vi "FrontPanel-20220513-backup.vi"() -> ()   [LabVIEW 2019]
doc: "This VI controls the blindpanel type GHS-2T-1T-700 for a CryoFree DR. Automatization control is embedded in the blindpanel. Keys can be manipulated from within this VI."
uses:
  1. Sources/Lib/Lib.llb/ErrCodeStatusLkup.vi
  1. Sources/Lib/Lib.llb/Pfeiffer Vacuum.lvlib
  1. Sources/Lib/Lib.llb/MView.lvlib
  1. Sources/Lib/Lib.llb/Busy PopUp.lvlib
  shared/FP-TC-Shared/FP-TC-Shared.lvclass
panel:
  out "VIRef":T1 {"Array DataType" format="%.0x"; "WaveForm Type" format="%.0x"; "RefNum Type" format="%.0x"; "DataType" format="%.0x"}
  out "ControlNames":string[](array[string])
  in  "Toolbar":enum32{"Page 1", "Page 2"}(tab)
  in  "Load config":bool
  in  "Save config":bool
  in  "Start":bool
  in  "Stop":bool
  out "V":string
  out "PT2 Data":dbl[](array[numeric])
  in  "Restart PT on Error?":bool
  in  "Attempts":u16=6
  in  "Time delay":u16=60 format="%.0f s"
  out "Error Log":string[][](table)
  in  "Error panel":enum32{"Page 1"}(tab)
  out "PT2 error":errorcluster
  out "MG error":errorcluster
  out "PT1 error":errorcluster
  out "FP error":errorcluster
  out "PT1 Data":dbl[](array[numeric])
  in  "Main Panel":enum32{"Page 1", "Page 2"}(tab)
  out "PC":sgl
  out "P1":sgl format="%.1f"
  out "P2":sgl format="%.1f"
  out "P3":sgl format="%.1f"
  out "P4":sgl format="%.1f"
  out "P5":sgl format="%.1f"
  out "P6":sgl format="%.1f"
  out "P7":sgl format="%.1f"
  out "Flow":sgl format="%#_4f"
  out "P5 alarm":bool
  out "Pstill (P8)":dbl format="%.1e"
  in  "Main Panel":T2(tab)
  out "String 2":string
  out "String 4":string
  out "String":string
  out "String 3":string
  out "Mode":u16(ring) items=["AUTO MODE OFF", "START", "CONDENSING 3He", "CONDENSING 4He", "NORMAL CIRCULATION", "RECOVERY OF THE MIXTURE", "RECOVERY: BLOCKAGE OR OVERPRESSURE"]
  out "FLOW":sgl format="%#_3f"
  out "P5":sgl
  out "P4":sgl
  out "P3":sgl
  out "P1":sgl
  out "P2":sgl
  out "3He":sgl(slide) min=0 max=2 scale=0.0..2000.0 scale format="%.2f"
  out "4He":sgl(slide) min=0 max=2 scale=0.0..2000.0 scale format="%.2f"
  out "Panel ID":string
  in  "FP type":enum32{"OLD", "NEW"}(tab)
  in  "Buttons":T3
  out "LEDs":T4
  in  "Buttons 2":T3
  out "LEDs 2":T5
  out "PC":sgl
  in  "PT Start 2":bool
  in  "PT_stop 2":bool
  in  "PT2 Plots Select":T6
  out "PT2 Status":cluster{"Time":dbl[], "Value":dbl[]}[](graph)
  in  "PT_ResetValues 2":bool
  out "PT Error Code 2":i32 caption="PT Error Code"
  out "PT Error 2":string="NO ERROR" caption="PT Error"
  out "P High":cluster{dbl, dbl, dbl, dbl}(slide) scale=150.0..450.0
  out "P Low":cluster{dbl, dbl, dbl, dbl}(slide) scale=0.0..300.0
  out "P_avg 2":cluster{"Low":dbl, "High":dbl} caption="Average pressure"
  out "Helium":cluster{dbl, dbl, dbl, dbl}(slide) scale=0.0..95.0
  out "Water In":cluster{dbl, dbl, dbl, dbl}(slide) scale=0.0..35.0
  out "Water Out":cluster{dbl, dbl, dbl, dbl}(slide) scale=0.0..60.0
  out "PT Status":u16(ring) items=["Compressor OFF", "Compressor ON", ""]
  out "Motor":cluster{dbl, dbl}(slide) scale=0.0..30.0
  out "Oil":cluster{dbl, dbl, dbl, dbl}(slide) scale=0.0..60.0
  in  "PT1 Plots Select":T6
  out "PT1 Status 2":cluster{"Time":dbl[], "Value":dbl[]}[](graph)
  out "P Low":cluster{dbl, dbl, dbl, dbl}(slide) scale=0.0..300.0
  out "P High":cluster{dbl, dbl, dbl, dbl}(slide) scale=150.0..450.0
  out "P_avg":cluster{"Low":dbl, "High":dbl} caption="Average pressure"
  out "Motor":cluster{dbl, dbl}(slide) scale=0.0..30.0
  out "Oil":cluster{dbl, dbl, dbl, dbl}(slide) scale=0.0..60.0
  out "Helium":cluster{dbl, dbl, dbl, dbl}(slide) scale=0.0..95.0
  out "Water Out":cluster{dbl, dbl, dbl, dbl}(slide) scale=0.0..60.0
  out "Water In":cluster{dbl, dbl, dbl, dbl}(slide) scale=0.0..35.0
  out "PT Error Code":i32
  out "PT Error":string="NO ERROR"
  in  "PT_ResetValues":bool
  in  "PT Start":bool
  in  "PT_stop":bool
  out "PT Status":u16(ring) items=["Compressor OFF", "Compressor ON", ""]
  in  "MG Plots Select":T6
  in  "FP Plots Select":T6
  out "MaxiGauge":cluster{"Time":dbl[], "Value":dbl[]}[](graph)
  out "Front Panel":cluster{"Time":dbl[], "Value":dbl[]}[](graph)
  in  "Boolean 2":bool
  out "PT2 port":u16
  out "PT1 port":u16
  out "MG port":refnum<visa-resource-name>="COM4" caption="Port number"
  out "FP port":refnum<visa-resource-name>="COM3" caption="Port number"
  out "ForceSave":bool
  in  "Button":u8
  out "SetControl":T7
  in  "S2":enum32{"Page 1"}(tab)
  in  "Reset Error 2":bool
  in  "S1":enum32{"Page 1"}(tab)
  in  "Reset Error":bool
  out "Cur Path":path
  in  "Side Panel":enum32{"Main", "Settings", "Advanced"}(tab)=enum."Settings"
  out "Maxigauge ID":string caption="ID"
  out "Panel response":string
  out "Sensors Status":T8={"String 8"="OK", "String 9"="OK", "String 10"="OK", "String 11"="OK", "String 12"="OK", "String 13"="OK"}
  in  "ADC scaling":T9={"P1"=2500.0, "P2"=2500.0, "P3"=2500.0, "P4"=2500.0, "P5"=2500.0, "P6"=2500.0, "P7"=2500.0, "Flow meter"=682.0, "PC"=10000.0} caption="Front panel ADC scaling factors" {"Flow meter" format="%#.4f"}
  in  "REC Settings":T10={"P6 low"=20, "P6 high"=1000, "P7 low"=20}
  in  "NCP5B Settings":cluster{"P6 low":u16}={"P6 low"=20}
  in  "NCP5 Settings":T10={"P6 low"=20, "P6 high"=1000, "P7 low"=20}
  in  "S1&2 Settings":cluster{"Enum":enum16{"OFF", "ON"}}
  in  "P5 Settings":cluster{"P6 low":u16, "P6 high":u16}={"P6 low"=20, "P6 high"=1000}
  out "REC limits":T11={"P5 warn"=20, "P5 rec"=20, "P5 res"=20}
  out "NCP5B limits":cluster{"P5 NC4":u16}={"P5 NC4"=20}
  out "NCP5 limits":T12={"P5 NC1"=20, "P5 NC2"=20, "P5 NC3"=20}
  out "S1&2 limits":cluster{"S1&S2":enum16{"OFF", "ON"}}
  out "P5 limits":cluster{"P5 C1":u16, "P5 C2":u16}={"P5 C1"=20, "P5 C2"=20}
  in  "P6&7 Settings":T13={"P6 low"=20, "P6 high"=1600, "P7 low"=20, "P7 high"=1610}
  out "P6&7 limits":T13={"P6 low"=20, "P6 high"=20, "P7 low"=20, "P7 high"=20}
  in  "SET VALUES":bool
  out "MG pressures":T14 {"Channel 1" format="%-7.2e mbar"; "Channel 1" format="%-7.2e mbar"; "Channel 1" format="%-7.2e mbar"; "Channel 1" format="%-7.2e mbar"; "Channel 1" format="%-7.2e mbar"; "Channel 1" format="%-7.2e mbar"}
  out "Cluster":T15={"String 2"="\"\"", "String 3"="", "String 4"="", "String 5"="", "String 6"="", "String 7"=""}
  in  "Log Options":T16={"Plot data "=TRUE, "Every1"=1.0, "Save to log"=TRUE, "Every  2"=1.0, "AVS_Path 2"=path "C:/LC Data/Data", "AVS_FName"="logFP", "Filename suffix"="_%Y-%m-%d-%H-%M-%S", "NewFevery"=7, "Time Units"=enum."Days", "Date Format"="%Y-%m-%d %H:%M:%S", "Averages"=4} caption="Data Logging \nOptions" {"Every  2" format="%#_g min"; "Every1" format="%#_g min"}
  in  "Configuration":T17={"FP port number"="COM3", "MG port number"="COM4", "PT1 Enabled?"=FALSE, "MG  channel P8"=65535, "Stop auto recovery if still is empty"=FALSE, "PT1 port number"="COM2", "MG Enabled?"=TRUE, "PT1 Address"=16, "S1 Enabled?"=FALSE, "S1 port"="COM2", "S2 Enabled?"=FALSE, "S2 port"="COM2", "Device address S1"=1, "Device address S2"=2, "PT1 Bauds"=115200, "PT2 Enabled?"=FALSE, "PT2 port number"="COM2", "PT2 Address"=16, "PT2 Bauds"=115200, "FP baud rate"=9600} {"PT2 Address" min=16 max=126 step=1; "MG  channel P8" items=["Channel 1", "Channel 2", "Channel 3", "Channel 4", "Channel 5", "Channel 6"]; "PT1 Address" min=16 max=126 step=1}
  in  "Type":enum32{"Wet", "CF"}(radio)=enum."CF"
  in  "Panel Layout":enum32{"OLD", "NEW"}(ring)=enum."NEW"
  out "RAW ADC Values 2":dbl[](array[numeric]) caption="Converted ADC Values"
  in  "SendCMD":bool caption="Send"
  out "Response":string
  in  "Command":string
  out "SP reached? 2":bool
  in  "Cond1":bool
  in  "Delay Time":u32=30 caption="For a time delay of" format="%.0f min"
  in  "MG  channel":u16(ring)=65535 caption="MaxiGauge" items=["Channel 1", "Channel 2", "Channel 3", "Channel 4", "Channel 5", "Channel 6"]
  out "SP reached? 3":bool
  in  "P threshold":dbl=0.0005 caption="<" format="%#_2g mbar"
  in  "Cond2":bool
  out "SP reached?":bool
  out "Delay Timer":u32=10 caption="Timer" format="%<%M:%S>t"
  in  "EnableAutoCond":bool caption="Start"
  out "VI path":string
  out "RAW ADC Values":i32[](array[numeric])
  in  "Autoconf":bool caption="Autoconfigure"
  out "MG Data":dbl[](array[numeric]) format="%.3e"
  out "FP Data":sgl[](array[numeric]) format="%.2f"
  out "FP Status bits":u32[](array[numeric])
  out "Attempts Counter":u16
  # "Error log"
  # "Front panel status"
  # "MaxiGauge status"
  # "Pulse Tube 1 status"
  # "Pulse Tube 2 status"
  # "Leiden Cryogenics"
  # "to \nair"
  # "N.C."
  # "from\novc"
  # "from\nivc"
  # "from still"
  # "to 3He\nin-1"
  # "to 3He\nin-2"
  # "P8"
  # "AUX 1"
  # "BYPASS"
  # "MIXTURE\nCOMPRESSOR"
  # "M2"
  # "P6"
  # "M3"
  # "M1"
  # "AUX PORT-1"
  # "P7"
  # "TRAP"
  # "AUX TRAP"
  # "To \nAir"
  # "From\nIVC"
  # "From Still"
  # "To 3He\nin-1"
  # "To 3He\nin-2"
  # "To \nAir"
  # "N.C."
  # "from\novc"
  # "from\nivc"
  # "from still"
  # "to 3He\nin-1"
  # "to 3He\nin-2"
  # "Leiden Cryogenics"
  # "to \nair"
  # "N.C."
  # "from\novc"
  # "from\nivc"
  # "from still"
  # "to 3He\nin-1"
  # "to 3He\nin-2"
  # "P8"
  # "M2"
  # "P6"
  # "M3"
  # "TRAP"
  # "AUX TRAP"
  # "M1"
  # "AUX PORT-1"
  # "P7"
  # "AUX 1"
  # "To \nAir"
  # "From\nIVC"
  # "From Still"
  # "To 3He\nin-1"
  # "to 3He\nin-1"
  # "To 3He\nin-2"
  # "to \nair"
  # "N.C."
  # "from\novc"
  # "from\nivc"
  # "from still"
  # "to 3He\nin-2"
  # "Pulse Tube 1"
  # "Pulse Tube 2"
  # "Front Panel"
  # "MaxiGauge"
  # "Turbo2 (S2)"
  # "Turbo1 (S1)"
  # "MaxiGauge"
  # "#"
  # "NAME"
  # "PRESSURE"
  # "STATUS"
  # "1"
  # "2"
  # "3"
  # "4"
  # "5"
  # "6"
  # "Automatic mode pressure limits"
  # "Warning: These values influence the operation of the GHS in automatic mode. Please refer to the operation manual and consult with Leiden Cryogenics before changing them."
  # "NAME"
  # "FW"
  # "NEW"
  # "DESCRIPTION"
  # "Stop condensing 4He"
  # "Stop recovering 4He"
  # "Stop condensing 3He"
  # "Stop recovering 3He"
  # "Condensing->open 12"
  # "Condensing->close 9/12"
  # "Condensing->run S1&S2"
  # "NC->open second line"
  # "NC->start MC"
  # "NC->open aux. trap"
  # "NC->stop MC, close 7"
  # "All->P5 alarm"
  # "All->switch to recovery"
  # "All->reset"
  # "Front panel ADC scaling factors"
  # "Data Logging and Plotting"
  # "Front Panel"
  # "MaxiGauge"
  # "Pulse Tube 1"
  # "Pulse Tube 2"
  # "Turbo 1 (S1) (Pfeiffer HiPACE only)"
  # "Turbo2 (S2) (Pfeiffer HiPACE only)"
  # "Automatic condensing"
  # "Start condensing when"
  # "and wait"
  # "Send command to Front Panel"
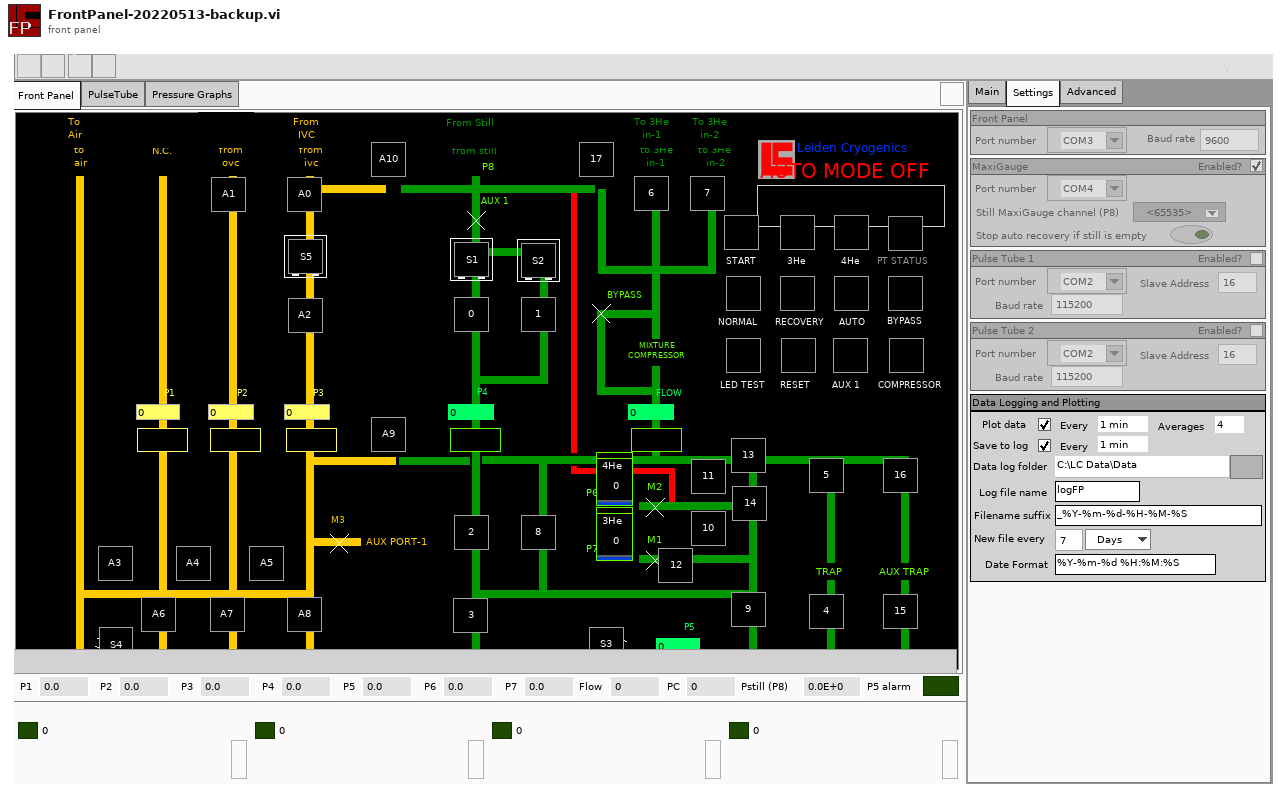
[diagram p1: front panel]
types:
  T1 = cluster{"Control Ref ID":refnum<vi>[], "Full Name":string[], "ClassID":enum16{"<Null>", "1", "2", "Generic", "Decoration", "Text", "Control", "ColorBox", "Boolean", "RefNum", "Variant", "Path", "ListBox", "Table", "Array", "Picture", "ActiveXContainer", "Numeric", "Digital", "NamedNumeric", "ColorRamp", "Slide", "GraphOrChart", "WaveformChart", "WaveformGraph", "IntensityChart", "IntensityGraph", "String", "IOName", "ComboBox", "Cluster", "Panel", "Knob", "NumWithScale", "Ring", "Enum", "GObject", "Plot", "Cursor", "NumericText", "Scale", "ColorScale", "GraphScale", "ColorGraphScale", "TypedRefNum", "OldKnobScale", "MCListbox", "MeasureData", "BVTag", "DAQName", "VISAName", "IVIName", "SlideScale", "TabControl", "Page", "TabArrayTabControl", "ConPane", "57", "58", "59", "60", "61", "62", "63", "64", "SubPanel", "TreeControl", "67", "68", "69", "70", "71", "72", "73", "74", "75", "SplitterBar"}[], "Short Name":string[], "DataType":enum8{"<Null>", "I8", "I16", "I32", "I64", "U8", "U16", "U32", "U64", "SGL", "DBL", "EXT", "CSG", "CDB", "CXT", "0x0F", "0x10", "0x11", "0x12", "0x13", "0x14", "Enum U8", "Enum U16", "Enum U32", "Enum U64", "SGL PQ", "DBL PQ", "EXT PQ", "CSG PQ", "CDB PQ", "CXT PQ", "0x1F", "0x20", "Boolean", "0x22", "0x23", "0x24", "0x25", "0x26", "0x27", "0x28", "0x29", "0x2A", "0x2B", "0x2C", "0x2D", "0x2E", "0x2F", "String", "0x31", "Path", "Pict", "0x34", "0x35", "0x36", "DAQ", "0x38", "0x39", "0x3A", "0x3B", "0x3C", "0x3D", "0x3E", "0x3F", "Array", "0x41", "0x42", "0x43", "0x44", "0x45", "0x46", "0x47", "0x48", "0x49", "0x4A", "0x4B", "0x4C", "0x4D", "0x4E", "0x4F", "Cluster", "0x51", "0x52", "Variant", "Waveform", "0x55", "0x56", "0x57", "0x58", "0x59", "0x5A", "0x5B", "0x5C", "0x5D", "0x5E", "0x5F", "0x60", "0x61", "0x62", "0x63", "0x64", "0x65", "0x66", "0x67", "0x68", "0x69", "0x6A", "0x6B", "0x6C", "0x6D", "0x6E", "0x6F", "Refnum"}[], "RefNum Type":enum8{"Generic", "Datalog File Refnum", "Byte Stream File Refnum", "Device Refnum", "Occurence Refnum", "TCP Connection Refnum", "VISA Refnum (Obsolete)", "Automation Renum", "VI Server Refnum", "Menu Refnum", "IVI Refnum (Obsolete)", "IMAQ Session", "0x0C", "Datasocket Refnum", "VISA Resource", "IVI Logical Name", "UDP Connection Refnum", "Notifier Refnum", "Queue Refnum", "IrDA Refnum", "Hardware Plugin Refnum", "Hardware Plugin Tag Refnum", "DAQmx Refnum", "Event Registration Refnum", ".NET Refnum", "User Event Refnum", "0x1A", "Event Callback", "0x1C", "0x1D", "Only Used Internal to LabVIEW", "Bluetooth", "Data Value References", "RT FIFO", "TDM Streaming"}[], "WaveForm Type":enum8{"<Not a Waveform Type>", "0x01", "Analog 16-bit signed", "Analog Double-Precision", "0x04", "Analog Single Precision", "Timestamp", "Digital Data", "Digital Waveform", "Dynamic Data", "Analog Extended-Precision", "Analog 8-bit unsigned", "Analog 16-bit unsigned", "Analog 32-bit unsigned", "Analog 8-bit signed", "Analog 32-bit signed", "Analog Complex Single-Precision", "Analog Complex Double-Precision", "Analog Complex Extended Precision", "Analog 64-bit signed", "Analog 64-bit unsigned"}[], "Parent":i32[], "Array DataType":enum8{"<Null>", "I8", "I16", "I32", "I64", "U8", "U16", "U32", "U64", "SGL", "DBL", "EXT", "CSG", "CDB", "CXT", "0x0F", "0x10", "0x11", "0x12", "0x13", "0x14", "Enum U8", "Enum U16", "Enum U32", "Enum U64", "SGL PQ", "DBL PQ", "EXT PQ", "CSG PQ", "CDB PQ", "CXT PQ", "0x1F", "0x20", "Boolean", "0x22", "0x23", "0x24", "0x25", "0x26", "0x27", "0x28", "0x29", "0x2A", "0x2B", "0x2C", "0x2D", "0x2E", "0x2F", "String", "0x31", "Path", "Pict", "0x34", "0x35", "0x36", "DAQ", "0x38", "0x39", "0x3A", "0x3B", "0x3C", "0x3D", "0x3E", "0x3F", "Array", "0x41", "0x42", "0x43", "0x44", "0x45", "0x46", "0x47", "0x48", "0x49", "0x4A", "0x4B", "0x4C", "0x4D", "0x4E", "0x4F", "Cluster", "0x51", "0x52", "Variant", "Waveform", "0x55", "0x56", "0x57", "0x58", "0x59", "0x5A", "0x5B", "0x5C", "0x5D", "0x5E", "0x5F", "0x60", "0x61", "0x62", "0x63", "0x64", "0x65", "0x66", "0x67", "0x68", "0x69", "0x6A", "0x6B", "0x6C", "0x6D", "0x6E", "0x6F", "Refnum"}[], "Owning VI":refnum<vi>[], "Active?":bool[]}
  T2 = enum32{"Front Panel", "PulseTube", "Pressure Graphs"}
  T3 = cluster{"baux2":bool, "bBypass":bool, "b15":bool, "b16":bool, "NC 0":bool, "baux1":bool, "b4":bool, "NC 1":bool, "b5":bool, "breset":bool, "NC 2":bool, "b9":bool, "b14":bool, "NC 3":bool, "b13":bool, "bledtest":bool, "NC 4":bool, "b12":bool, "b10":bool, "NC 5":bool, "b11":bool, "bA0":bool, "NC 9":bool, "b7":bool, "bS3":bool, "NC 12":bool, "b6":bool, "b17":bool, "NC 13":bool, "b8":bool, "b1":bool, "NC 14":bool, "bS2":bool, "b3":bool, "NC 15":bool, "b2":bool, "b0":bool, "NC 16":bool, "bS1":bool, "bA9":bool, "NC 17":bool, "bA8":bool, "bA2":bool, "NC 6":bool, "bs5":bool, "bA10":bool, "NC 7":bool, "bstart":bool, "bA5":bool, "NC 8":bool, "bA7":bool, "bA1":bool, "NC 10":bool, "bauto":bool, "bA4":bool, "NC 11":bool, "bA6":bool, "bS4":bool, "NC 18":bool, "bA3":bool, "b3he":bool, "b4he":bool, "bnorm":bool, "brecov":bool}
  T4 = cluster{"COMPR/AUX 2":bool, "BYPASS":bool, "15":bool, "16":bool, "NC 0":bool, "AUX 1":bool, "4":bool, "NC 1":bool, "5":bool, "RESET":bool, "NC 2":bool, "9":bool, "14":bool, "NC 3":bool, "13":bool, "LED TEST":bool, "NC 4":bool, "12":bool, "10":bool, "NC 5":bool, "11":bool, "A0":bool, "NC 12":bool, "7":bool, "S3":bool, "NC 13":bool, "6":bool, "17":bool, "NC 14":bool, "8":bool, "1":bool, "NC 15":bool, "S2":bool, "3":bool, "NC 16":bool, "2":bool, "0":bool, "NC 17":bool, "S1":bool, "A9":bool, "NC 6":bool, "A8":bool, "A2":bool, "NC 7":bool, "S5":bool, "A10":bool, "NC 8":bool, "START":bool, "A5":bool, "NC 9":bool, "A7":bool, "A1":bool, "NC 10":bool, "AUTO":bool, "A4":bool, "NC 11":bool, "A6":bool, "S4":bool, "NC 18":bool, "A3":bool, "3He":bool, "4He":bool, "NORMAL":bool, "RECOVERY":bool, "PT STATUS":bool}
  T5 = cluster{"COMPR/AUX 2":bool, "BYPASS":bool, "15":bool, "16":bool, "AUX 1":bool, "AUX 1":bool, "4":bool, "AUX 2":bool, "5":bool, "RESET":bool, "AUX 3":bool, "9":bool, "14":bool, "NC 3":bool, "13":bool, "LED TEST":bool, "NC 4":bool, "12":bool, "10":bool, "NC 5":bool, "11":bool, "A0":bool, "NC 12":bool, "7":bool, "S3":bool, "NC 13":bool, "6":bool, "17":bool, "NC 14":bool, "8":bool, "1":bool, "NC 15":bool, "S2":bool, "3":bool, "NC 16":bool, "2":bool, "0":bool, "NC 17":bool, "S1":bool, "A9":bool, "NC 6":bool, "A8":bool, "A2":bool, "NC 7":bool, "S5":bool, "A10":bool, "NC 8":bool, "START":bool, "A5":bool, "NC 9":bool, "A7":bool, "A1":bool, "NC 10":bool, "AUTO":bool, "A4":bool, "NC 11":bool, "A6":bool, "S4":bool, "NC 18":bool, "A3":bool, "3He":bool, "4He":bool, "NORMAL":bool, "RECOVERY":bool, "PT STATUS":bool}
  T6 = cluster{"Boolean":bool, "Boolean 2":bool, "Boolean 3":bool, "Boolean 4":bool, "Boolean 5":bool, "Boolean 6":bool, "Boolean 7":bool, "Boolean 8":bool}
  T7 = cluster{"Name":string, "Scalar":string, "Array":string[][]}
  T8 = cluster{"String 8":string, "String 9":string, "String 10":string, "String 11":string, "String 12":string, "String 13":string}
  T9 = cluster{"P1":dbl, "P2":dbl, "P3":dbl, "P4":dbl, "P5":dbl, "P6":dbl, "P7":dbl, "Flow meter":dbl, "PC":dbl}
  T10 = cluster{"P6 low":u16, "P6 high":u16, "P7 low":u16}
  T11 = cluster{"P5 warn":u16, "P5 rec":u16, "P5 res":u16}
  T12 = cluster{"P5 NC1":u16, "P5 NC2":u16, "P5 NC3":u16}
  T13 = cluster{"P6 low":u16, "P6 high":u16, "P7 low":u16, "P7 high":u16}
  T14 = cluster{"Channel 1":dbl, "Channel 1":dbl, "Channel 1":dbl, "Channel 1":dbl, "Channel 1":dbl, "Channel 1":dbl}
  T15 = cluster{"String 2":string, "String 3":string, "String 4":string, "String 5":string, "String 6":string, "String 7":string}
  T16 = cluster{"Plot data ":bool, "Every1":dbl, "Save to log":bool, "Every  2":dbl, "AVS_Path 2":path, "AVS_FName":string, "Filename suffix":string, "NewFevery":u32, "Time Units":enum16{"Minutes", "Hours", "Days"}, "Date Format":string, "Averages":i32}
  T17 = cluster{"FP port number":refnum<visa-resource-name>, "MG port number":refnum<visa-resource-name>, "PT1 Enabled?":bool, "MG  channel P8":u16, "Stop auto recovery if still is empty":bool, "PT1 port number":refnum<visa-resource-name>, "MG Enabled?":bool, "PT1 Address":u8, "S1 Enabled?":bool, "S1 port":refnum<visa-resource-name>, "S2 Enabled?":bool, "S2 port":refnum<visa-resource-name>, "Device address S1":u8, "Device address S2":u8, "PT1 Bauds":u32, "PT2 Enabled?":bool, "PT2 port number":refnum<visa-resource-name>, "PT2 Address":u8, "PT2 Bauds":u32, "FP baud rate":u32}
  T18 = cluster{"error":bool, "code":i32, "source":string}
  T19 = cluster{"Dict. Var":u16, "Description":string, "Values":i32[]}[]
  T20 = cluster{"[3]":dbl, "[3]":dbl, "[3]":dbl, "Values[3] 2":dbl}
  T21 = cluster{"[1]":dbl, "[1]":dbl, "[1]":dbl, "Values[1] 2":dbl}
  T22 = cluster{"Values[0]":dbl, "Values[0]":dbl, "Values[0]":dbl, "Values[0] 2":dbl}
  T23 = cluster{"error":bool, "code":i32, "error source":string}
  T24 = cluster{"sensor status info[0]":string, "sensor status info[1]":string, "sensor status info[2]":string, "sensor status info[3]":string, "sensor status info[4]":string, "sensor status info[5]":string}
  T25 = cluster{"Filterred[0]":dbl, "Filterred[1]":dbl, "Filterred[2]":dbl, "Filterred[3]":dbl, "Filterred[4]":dbl, "Filterred[5]":dbl}
  T26 = cluster{"FP Data[0]":sgl, "FP Data[1]":sgl, "FP Data[2]":sgl, "FP Data[3]":sgl, "FP Data[4]":sgl, "FP Data[5]":sgl, "FP Data[6]":sgl, "FP Data[7]":sgl, "FP Data[8]":sgl}
  T27 = enum32{"Page Enabled", "Page Disabled", "Page Disabled & Grayed"}
  T28 = enum32{"invalid app kind", "Development System", "Run Time System", "Student Edition", "Embedded LabVIEW", "Evaluation", "Custom"}
  T29 = cluster{"array of 4 x 16 bit unsigned[0]":u16, "array of 4 x 16 bit unsigned[1]":u16, "array of 4 x 16 bit unsigned[2]":u16, "array of 4 x 16 bit unsigned[3]":u16}
  T30 = cluster{"array of 2 x 16 bit unsigned[0]":u16, "array of 2 x 16 bit unsigned[1]":u16}
  T31 = cluster{"array of 3 x 16 bit unsigned[0]":u16, "array of 3 x 16 bit unsigned[1]":u16, "array of 3 x 16 bit unsigned[2]":u16}
  T32 = cluster{"Array[0]":string, "Array[1]":string, "Array[2]":string, "Array[3]":string, "Array[4]":string, "Array[5]":string}
  T33 = typedef "LVRectTypeDef.ctl" = cluster{"Left":i16, "Top":i16, "Right":i16, "Bottom":i16}
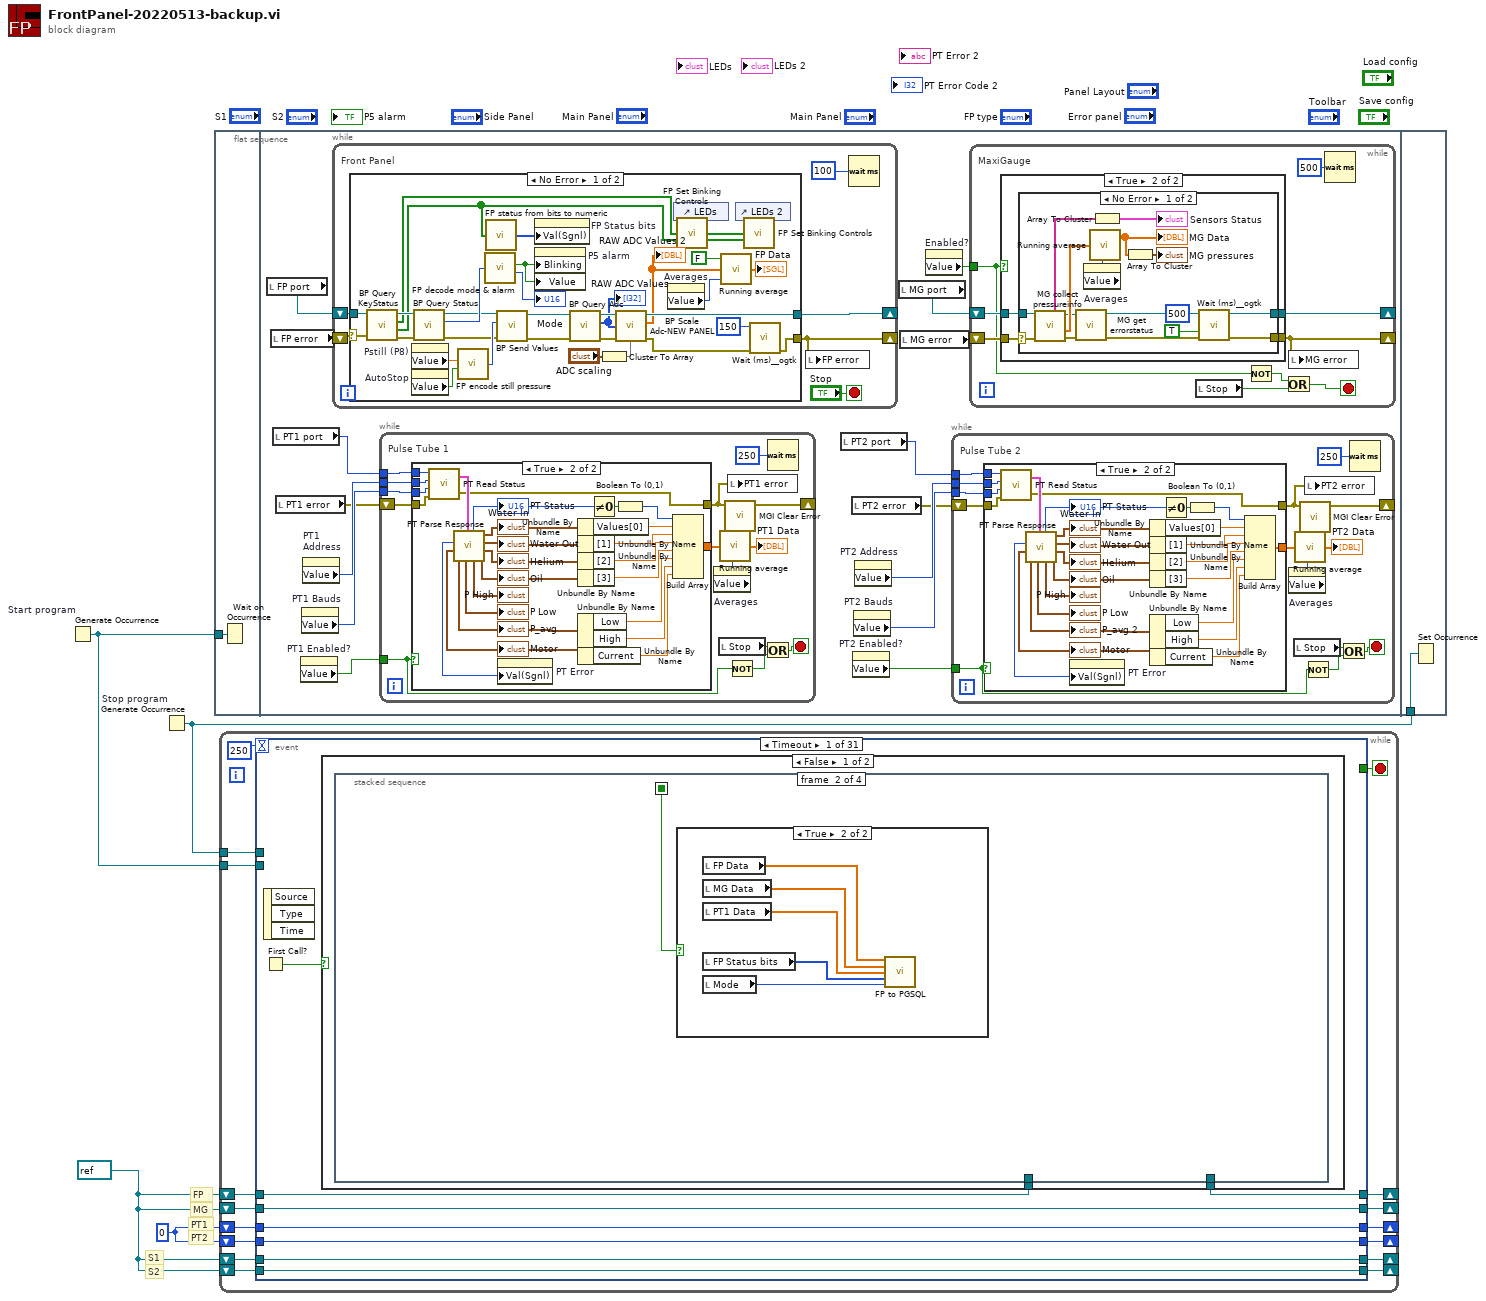
[diagram p0: block diagram]
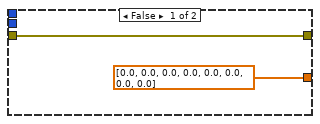
[diagram p2: hidden frame]
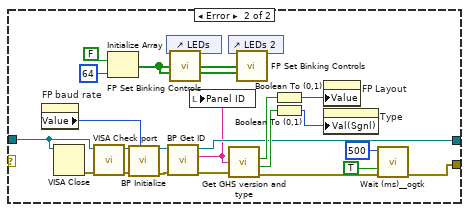
[diagram p3: hidden frame]
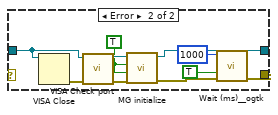
[diagram p5: hidden frame]
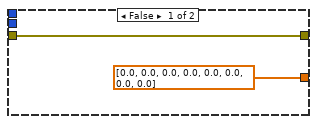
[diagram p6: hidden frame]
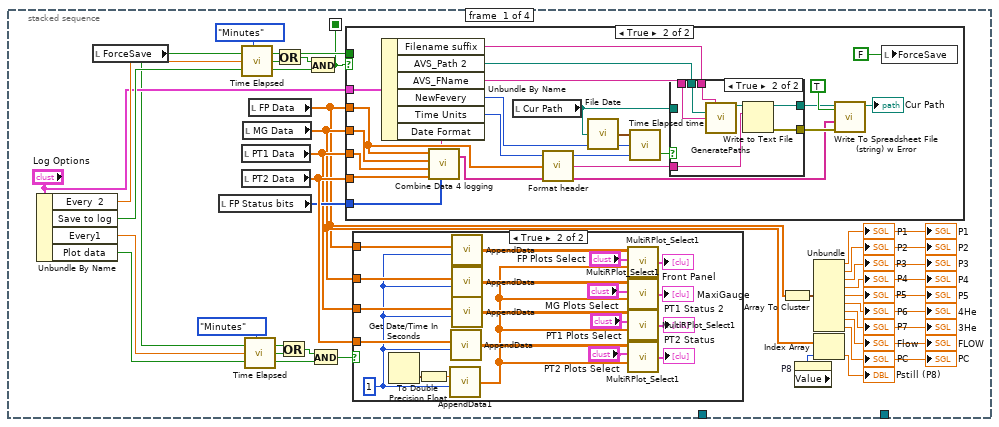
[diagram p7: hidden frame]
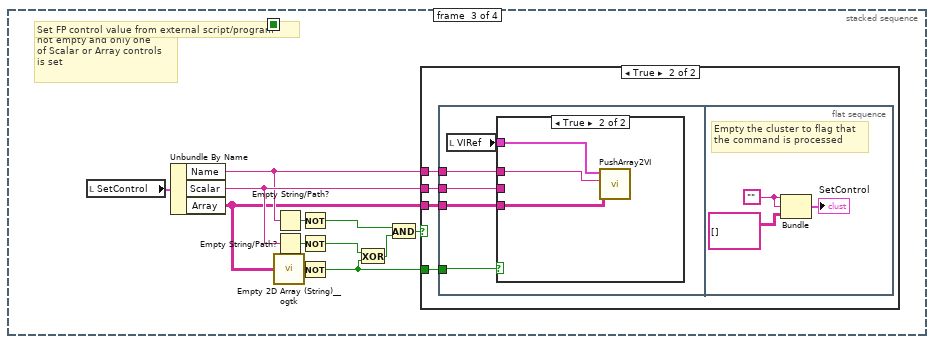
[diagram p12: hidden frame]
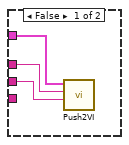
[diagram p14: hidden frame]
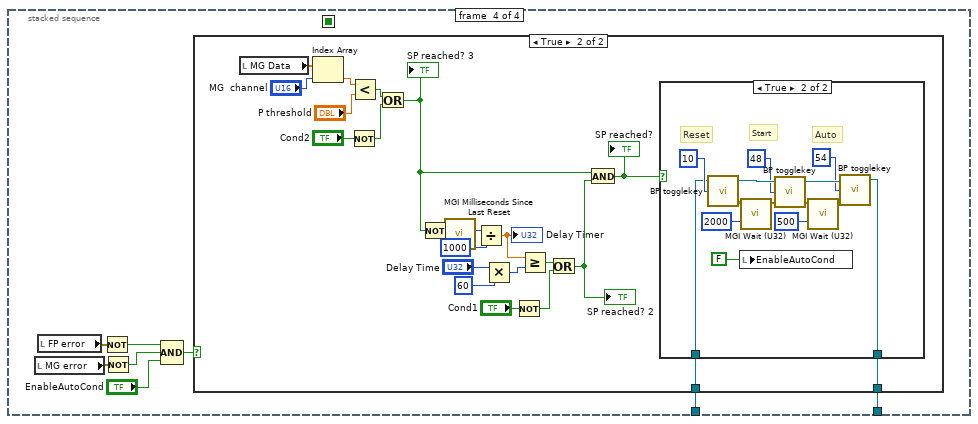
[diagram p15: hidden frame]
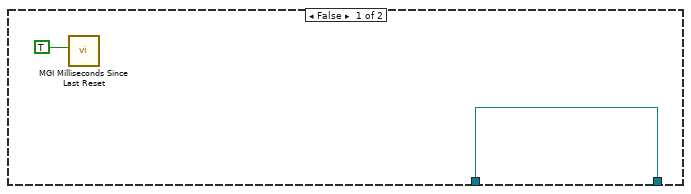
[diagram p16: hidden frame]
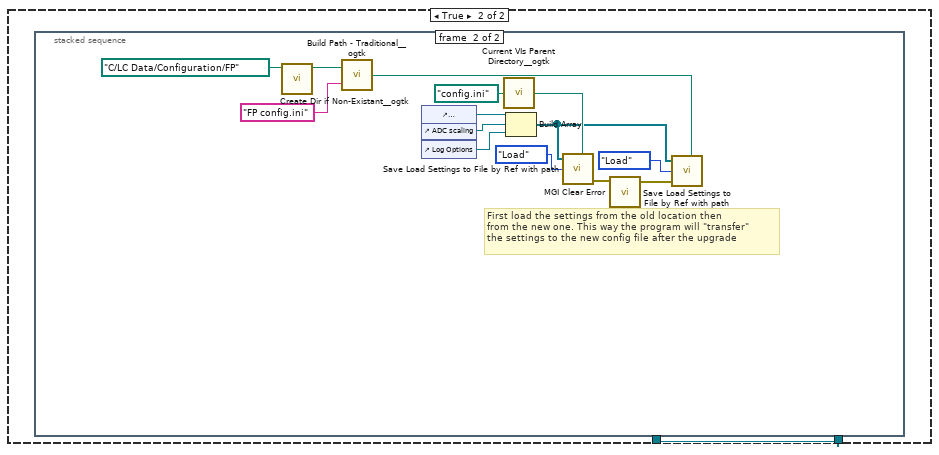
[diagram p18: hidden frame]
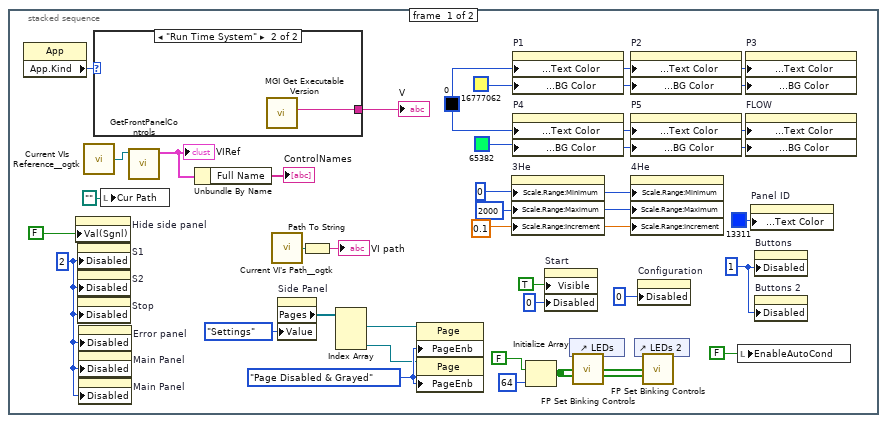
[diagram p19: hidden frame]
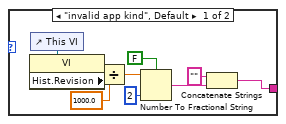
[diagram p20: hidden frame]
diagram:
  w1 = u8 0 ("x+1")
  w2 = refnum<visa-resource-name> refnum ("PT port")
  # "S2"
  # "S1"
  # "MG"
  # "PT1"
  # "PT2"
  # "FP"
  n1 = Generate Occurrence "Start program"() -> (w4:refnum<k4>)
  n2 = Generate Occurrence "Stop program"() -> (w3:refnum<k4>)
  n3 = flat-sequence {
    tunnel: w4 -> [w5]
    tunnel: w3 -> [w204]
    frame #0 {
      n4 = Wait on Occurrence(2:w5) -> ()  [unwired: 2 in, 1 out]
    }
    frame #1 {
      n5 = local read "FP port"() -> (w11:refnum<visa-resource-name>)
      n6 = local read "FP error"() -> (w16:errorcluster)
      n7 = local read "PT1 port"() -> (w7:u16)
      n8 = local read "PT1 error"() -> (w8:errorcluster)
      n9 = property on="PT1 Enabled?" class="Bool (strict)"() -> ("Value"=w19:bool)  [unwired: 2 in, 2 out]
      n10 = property on="PT1 Bauds" class="DigNum (strict)"() -> ("Value"=w17:u32)  [unwired: 2 in, 2 out]
      n11 = property on="PT1 \nAddress" class="DigNum (strict)"() -> ("Value"=w20:u8)  [unwired: 2 in, 2 out]
      n12 = while {
        shift-right: [w66] -> _
        shift-left: w16 -> [w67]
        shift-right: [w64] -> _
        shift-left: w11 -> [w65]
        stop <- "Stop" stop-if-true
        # "Front Panel"
        n13 = case shown="No Error" w67 {
          selector: w67 -> [w97 _]
          tunnel: [w78 w111] -> w64
          tunnel: [w76 w109] -> w66
          tunnel: w65 -> [w98 w112]
          frame No Error {
            n14 = call "BP Query KeyStatus.vi"("error in"=w97, "FrontPanel port"=w98) -> ("error out"=w86:T18, "Button states"=w69:bool[], "Blinking States"=w70:bool[], "FrontPanel port"=w87:refnum<visa-resource-name>)  [unwired: 2 in]
            n15 = property on="Pstill (P8)" class="DigNum (strict)"() -> ("Value"=w88:dbl)  [unwired: 2 in, 2 out]
            n16 = property on="AutoStop" class="Bool (strict)"() -> ("Value"=w89:bool)  [unwired: 2 in, 2 out]
            n17 = call "BP Query Status.vi"("error in"=w86, "FrontPanel port"=w87) -> ("error out"=w91:T18, "status word (32 bit unsigned)"=w94:u32, "FrontPanel port"=w92:refnum<visa-resource-name>)  [unwired: 3 in]
            n18 = call "FP encode still pressure.vi"("Value 2"=w89, "Value"=w88) -> ("Numeric"=w93:u16)  [unwired: 4 in]
            n19 = call "FP decode mode & alarm.vi"("status word (32 bit unsigned)"=w94) -> ("Boolean"=w90:bool, "Numeric"=→"Mode":u32)  [unwired: 4 in]
            n20 = call "FP status from bits to numeric.vi"("FP Status bits"=w69) -> ("FP status number"=w96:u32[])  [unwired: 4 in]
            n21 = call "BP Send Values.vi"("error in"=w91, "value to send"=w93, "FrontPanel port"=w92) -> ("error out"=w80:T18, "FrontPanel port"=w81:refnum<visa-resource-name>)  [unwired: 3 in]
            n22 = property on="FP Status bits" class="Arr (strict)"("Val(Sgnl)"=w96) -> ()  [unwired: 2 in, 2 out]
            n23 = property on="P5 alarm" class="Bool (strict)"("Blinking"=w90, "Value"=w90) -> ()  [unwired: 2 in, 2 out]
            n24 = call "BP Query Adc.vi"("error in"=w80, "FrontPanel port"=w81) -> ("error out"=w77:T18, "array of 8(9) x 16 bit signed"=w72:i32[], "FrontPanel port"=w78:refnum<visa-resource-name>)  [unwired: 3 in]
            "RAW ADC Values" <- w72
            n25 = Cluster To Array(cluster="ADC scaling") -> (array=w79:dbl[])
            n26 = call "BP Scale Adc-NEW PANEL.vi"("input array scaling factors,8(9) x 16 bit uint"=w79, "input array 8(9) x 16bit uint"=w72) -> ("output array 8(9) x single prec. incl flow"=w71:sgl[])  [unwired: 4 in, 1 out]
            "RAW ADC Values 2" <- w71
            n27 = property on="Averages" class="DigNum (strict)"() -> ("Value"=w85:i32)  [unwired: 2 in, 2 out]
            n28 = control-ref of="LEDs"() -> (w74:refnum<vi>)
            n29 = call "FP Set Binking Controls.vi"("Cluster in"=w74, "Array of blinking states"=w70, "Array of relais states"=w69) -> ()  [unwired: 13 in]
            n30 = call "Running average.vi"("Window Size"=w85, "New values"=w71, "Filter Zeroes? (T)"=FALSE) -> ("Filterred"=→"FP Data":dbl[])  [unwired: 1 in]
            n31 = control-ref of="LEDs 2"() -> (w73:refnum<vi>)
            n32 = call "FP Set Binking Controls.vi"("Cluster in"=w73, "Array of blinking states"=w70, "Array of relais states"=w69) -> ()  [unwired: 13 in]
            n33 = call <userlib>:"Wait (ms)__ogtk.vi"("error in (no error)"=w77, "milliseconds to wait"=u32 150) -> ("error out"=w76:errorcluster)  [unwired: 8 in, 1 out]
          }
          frame Error {
            n34 = property on="FP baud rate" class="DigNum (strict)"() -> ("Value"=w104:u32)  [unwired: 2 in, 2 out]
            n35 = VISA Close(VISA resource name=w112) -> (error out=w121:errorcluster)  [unwired: 1 in]
            n36 = call "VISA Check port.vi"("error in (no error)"=w121, "VISA Resource Name in"=w112) -> ("error out"=w120:errorcluster, "VISA Resource Name out"=w119:refnum<visa-resource-name>)  [unwired: 8 in]
            n37 = Initialize Array(FALSE, 64 ("dimension size")) -> (w99:bool[])
            n38 = call "BP Initialize.vi"("FP baud rate"=w104, "error in (no error)"=w120, "FrontPanel port"=w119) -> ("error out"=w118:errorcluster, "FrontPanel port"=w117:refnum<visa-resource-name>)  [unwired: 4 in]
            n39 = control-ref of="LEDs"() -> (w101:refnum<vi>)
            n40 = call "BP Get ID.vi"("error in (no error)"=w118, "FrontPanel port"=w117) -> ("error out"=w106:errorcluster, "Device ID string"=w110:string, "FrontPanel port"=w111:refnum<visa-resource-name>)  [unwired: 6 in, 1 out]
            n41 = call "FP Set Binking Controls.vi"("Cluster in"=w101, "Array of blinking states"=w99, "Array of relais states"=w99) -> ()  [unwired: 13 in]
            n42 = local write "Panel ID"(w110) -> ()
            n43 = control-ref of="LEDs 2"() -> (w100:refnum<vi>)
            n44 = call "Get GHS version and type.vi"("ID string"=w110, "error in (no error)"=w106) -> ("Panel Version"=w113:bool, "System Type"=w115:bool, "error out"=w105:errorcluster)  [unwired: 4 in]
            n45 = call "FP Set Binking Controls.vi"("Cluster in"=w100, "Array of blinking states"=w99, "Array of relais states"=w99) -> ()  [unwired: 13 in]
            n46 = Boolean To (0,1)(Boolean=w113) -> (0, 1=w114:i16)
            n47 = Boolean To (0,1)(Boolean=w115) -> (0, 1=w116:i16)
            n48 = property on="FP Layout" class="TabCtl (strict)"("Value"=w114) -> ()  [unwired: 2 in, 2 out]
            n49 = property on="Type" class="RadioBtnsControl (strict)"("Val(Sgnl)"=w116) -> ()  [unwired: 2 in, 2 out]
            n50 = call <userlib>:"Wait (ms)__ogtk.vi"("error in (no error)"=w105, "Wait on Error (FALSE)"=TRUE, "milliseconds to wait"=u32 500) -> ("error out"=w109:errorcluster)  [unwired: 7 in, 1 out]
          }
        }
        n51 = local write "FP error"(w66) -> ()
        n52 = Wait (ms)(milliseconds to wait=u32 100) -> ()  [unwired: 1 out]
      }
      n53 = while {
        tunnel: w7 -> [w174]
        tunnel: w20 -> [w173]
        tunnel: w19 -> [w164]
        tunnel: w17 -> [w170]
        shift-right: [w163] -> _
        shift-left: w8 -> [w169]
        stop <- w167 stop-if-true
        # "Pulse Tube 1"
        n54 = case shown="True" w164 {
          tunnel: [dbl[] [0.0, 0.0, 0.0, 0.0, 0.0, 0.0, 0.0, 0.0] w191] -> w175
          tunnel: w174 -> [_ w190]
          tunnel: w169 -> [w176 w189]
          tunnel: w173 -> [_ w188]
          tunnel: w170 -> [_ w183]
          tunnel: [w176 w182] -> w162
          frame False {
          }
          frame True {
            n55 = call "PT Read Status.vi"("error in (no error)"=w189, "Baud"=w183, "Slave Address"=w188, "Com Port #"=w190) -> ("error out"=w182:errorcluster, "Response"=w192:T19)
            n56 = call "PT Parse Response.vi"("Response"=w192) -> ("Oil temp"=w197:T20, "He temp"=w196:cluster{"[2]":dbl, "[2]":dbl, "[2]":dbl, dbl}, "Out water temp"=w195:T21, "In water temp"=w194:T22, "P_high"=→"P High":cluster{"[0]":dbl, "[0]":dbl, "[0]":dbl, dbl}, "Numeric"=w201:i32, "P_low"=→"P Low":cluster{"[1]":dbl, "[1]":dbl, "[1]":dbl, dbl}, "Average pressure"=w187:cluster{"Low":dbl, "High":dbl}, "Current"=w181:cluster{"Current":dbl, "Threshold":dbl}, "PT Error"=w193:i32)  [unwired: 1 in]
            "Oil" <- w197
            "Motor" <- w181
            "PT Status" <- w201
            "Water Out" <- w195
            "Water In" <- w194
            "Helium" <- w196
            "P_avg" <- w187
            n57 = property on="PT Error" class="DigNum (strict)"("Val(Sgnl)"=w193) -> ()  [unwired: 2 in, 2 out]
            n58 = Unbundle By Name(w194) -> ("Values[0]"=w184:dbl)
            n59 = Unbundle By Name(w195) -> ("[1]"=w200:dbl)
            n60 = Unbundle By Name(w196) -> ("[2]"=w199:dbl)
            n61 = Unbundle By Name(w197) -> ("[3]"=w198:dbl)
            n62 = Unbundle By Name(w187) -> ("Low"=w186:dbl, "High"=w185:dbl)
            n63 = Unbundle By Name(w181) -> ("Current"=w180:dbl)
            n64 = Not Equal To 0?(x=w201) -> (x != 0?=w202:bool)
            n65 = Boolean To (0,1)(Boolean=w202) -> (0, 1=w203:i16)
            n66 = Build Array(w203, w184, w200, w199, w198, w186, w185, w180) -> (w191:dbl[])
          }
        }
        n67 = property on="Averages" class="DigNum (strict)"() -> ("Value"=w172:i32)  [unwired: 2 in, 2 out]
        n68 = local read "Stop"() -> (w166:bool)
        n69 = call "Running average.vi"("Window Size"=w172, "New values"=w175) -> ("Filterred"=→"PT1 Data":dbl[])  [unwired: 2 in]
        n70 = call <userlib>:"MGI Clear Error.vi"("Error In"=w162) -> ("Error Out"=w163:errorcluster)  [unwired: 6 in]
        n71 = Not(x=w164) -> (.not. x?=w165:bool)
        n72 = local write "PT1 error"(w162) -> ()
        n73 = Or(x=w166, y=w165) -> (x .or. y?=w167:bool)
        n74 = Wait (ms)(milliseconds to wait=u32 250) -> ()  [unwired: 1 out]
      }
      n75 = local read "PT2 port"() -> (w6:u16)
      n76 = local read "PT2 error"() -> (w9:errorcluster)
      n77 = property on="PT2 Enabled?" class="Bool (strict)"() -> ("Value"=w13:bool)  [unwired: 2 in, 2 out]
      n78 = property on="PT2 Bauds" class="DigNum (strict)"() -> ("Value"=w12:u32)  [unwired: 2 in, 2 out]
      n79 = property on="PT2 Address" class="DigNum (strict)"() -> ("Value"=w14:u8)  [unwired: 2 in, 2 out]
      n80 = local read "MG port"() -> (w10:refnum<visa-resource-name>)
      n81 = local read "MG error"() -> (w15:errorcluster)
      n82 = property on="Enabled?" class="Bool (strict)"() -> ("Value"=w18:bool)  [unwired: 2 in, 2 out]
      n83 = while {
        tunnel: w6 -> [w33]
        tunnel: w14 -> [w32]
        tunnel: w13 -> [w23]
        tunnel: w12 -> [w29]
        shift-right: [w22] -> _
        shift-left: w9 -> [w28]
        stop <- w26 stop-if-true
        # "Pulse Tube 2"
        n84 = case shown="True" w23 {
          tunnel: [dbl[] [0.0, 0.0, 0.0, 0.0, 0.0, 0.0, 0.0, 0.0] w50] -> w34
          tunnel: w33 -> [_ w49]
          tunnel: w28 -> [w35 w48]
          tunnel: w32 -> [_ w47]
          tunnel: w29 -> [_ w42]
          tunnel: [w35 w41] -> w21
          frame False {
          }
          frame True {
            n85 = call "PT Read Status.vi"("error in (no error)"=w48, "Baud"=w42, "Slave Address"=w47, "Com Port #"=w49) -> ("error out"=w41:errorcluster, "Response"=w51:T19)
            n86 = call "PT Parse Response.vi"("Response"=w51) -> ("Oil temp"=w56:T20, "He temp"=w55:cluster{"[2]":dbl, "[2]":dbl, "[2]":dbl, dbl}, "Out water temp"=w54:T21, "In water temp"=w53:T22, "P_high"=→"P High":cluster{"[0]":dbl, "[0]":dbl, "[0]":dbl, dbl}, "Numeric"=w60:i32, "P_low"=→"P Low":cluster{"[1]":dbl, "[1]":dbl, "[1]":dbl, dbl}, "Average pressure"=w46:cluster{"Low":dbl, "High":dbl}, "Current"=w40:cluster{"Current":dbl, "Threshold":dbl}, "PT Error"=w52:i32)  [unwired: 1 in]
            "Oil" <- w56
            "Motor" <- w40
            "PT Status" <- w60
            "Water Out" <- w54
            "Water In" <- w53
            "Helium" <- w55
            "P_avg 2" <- w46
            n87 = property on="PT Error" class="DigNum (strict)"("Val(Sgnl)"=w52) -> ()  [unwired: 2 in, 2 out]
            n88 = Unbundle By Name(w53) -> ("Values[0]"=w43:dbl)
            n89 = Unbundle By Name(w54) -> ("[1]"=w59:dbl)
            n90 = Unbundle By Name(w55) -> ("[2]"=w58:dbl)
            n91 = Unbundle By Name(w56) -> ("[3]"=w57:dbl)
            n92 = Unbundle By Name(w46) -> ("Low"=w45:dbl, "High"=w44:dbl)
            n93 = Unbundle By Name(w40) -> ("Current"=w39:dbl)
            n94 = Not Equal To 0?(x=w60) -> (x != 0?=w61:bool)
            n95 = Boolean To (0,1)(Boolean=w61) -> (0, 1=w62:i16)
            n96 = Build Array(w62, w43, w59, w58, w57, w45, w44, w39) -> (w50:dbl[])
          }
        }
        n97 = property on="Averages" class="DigNum (strict)"() -> ("Value"=w31:i32)  [unwired: 2 in, 2 out]
        n98 = local read "Stop"() -> (w25:bool)
        n99 = call "Running average.vi"("Window Size"=w31, "New values"=w34) -> ("Filterred"=→"PT2 Data":dbl[])  [unwired: 2 in]
        n100 = call <userlib>:"MGI Clear Error.vi"("Error In"=w21) -> ("Error Out"=w22:errorcluster)  [unwired: 6 in]
        n101 = Not(x=w23) -> (.not. x?=w24:bool)
        n102 = local write "PT2 error"(w21) -> ()
        n103 = Or(x=w25, y=w24) -> (x .or. y?=w26:bool)
        n104 = Wait (ms)(milliseconds to wait=u32 250) -> ()  [unwired: 1 out]
      }
      n105 = while {
        tunnel: w18 -> [w123]
        shift-right: [w127] -> _
        shift-left: w15 -> [w126]
        shift-right: [w125] -> _
        shift-left: w10 -> [w128]
        stop <- w124 stop-if-true
        # "MaxiGauge"
        n106 = case shown="True" w123 {
          tunnel: w128 -> [w132 w136]
          tunnel: [w131 w135] -> w127
          tunnel: w126 -> [w131 w134]
          tunnel: [w132 w133] -> w125
          frame False {
          }
          frame True {
            n107 = case shown="No Error" w134 {
              selector: w134 -> [w143 _]
              tunnel: w136 -> [w151 w161]
              tunnel: [w137 w152] -> w135
              tunnel: [w150 w160] -> w133
              frame No Error {
                n108 = call "MG collect pressureinfo.vi"("error in"=w143, "MaxiGauge port"=w151) -> ("error out"=w148:T23, "sensor values"=w146:dbl[], "MaxiGauge port"=w142:refnum<visa-resource-name>, "sensor status info"=w141:string[])  [unwired: 4 in, 2 out]
                n109 = call "MG get errorstatus.vi"("error in"=w148, "MaxiGauge port"=w142) -> ("error out"=w138:T23, "MaxiGauge port"=w150:refnum<visa-resource-name>)  [unwired: 2 in, 2 out]
                n110 = property on="Averages" class="DigNum (strict)"() -> ("Value"=w145:i32)  [unwired: 2 in, 2 out]
                n111 = call "Running average.vi"("Window Size"=w145, "New values"=w146) -> ("Filterred"=w144:dbl[])  [unwired: 2 in]
                "MG Data" <- w144
                n112 = Array To Cluster(array=w141) -> (cluster=→"Sensors Status":T24)
                n113 = Array To Cluster(array=w144) -> (cluster=→"MG pressures":T25)
                n114 = call <userlib>:"Wait (ms)__ogtk.vi"("error in (no error)"=w138, "Wait on Error (FALSE)"=TRUE, "milliseconds to wait"=u32 500) -> ("error out"=w137:errorcluster)  [unwired: 7 in, 1 out]
              }
              frame Error {
                w156 = TRUE ("ID query")
                n115 = VISA Close(VISA resource name=w161) -> (error out=w159:errorcluster)  [unwired: 1 in]
                n116 = call "VISA Check port.vi"("error in (no error)"=w159, "VISA Resource Name in"=w161) -> ("error out"=w158:errorcluster, "VISA Resource Name out"=w157:refnum<visa-resource-name>)  [unwired: 8 in]
                n117 = call "MG initialize.vi"("error in (no error)"=w158, "MG query errorstatus"=w156, "ID query"=w156, "MaxiGauge port"=w157) -> ("error out"=w153:errorcluster, "MaxiGauge port"=w160:refnum<visa-resource-name>)  [unwired: 2 in, 1 out]
                n118 = call <userlib>:"Wait (ms)__ogtk.vi"("error in (no error)"=w153, "Wait on Error (FALSE)"=TRUE, "milliseconds to wait"=u32 1000) -> ("error out"=w152:errorcluster)  [unwired: 7 in, 1 out]
              }
            }
          }
        }
        n119 = local read "Stop"() -> (w129:bool)
        n120 = Not(x=w123) -> (.not. x?=w122:bool)
        n121 = Or(x=w122, y=w129) -> (x .or. y?=w124:bool)
        n122 = local write "MG error"(w127) -> ()
        n123 = Wait (ms)(milliseconds to wait=u32 500) -> ()  [unwired: 1 out]
      }
    }
    frame #2 {
      n124 = Set Occurrence(w204) -> ()
    }
  }
  n125 = while {
    shift-right: [w212] -> _
    shift-left: w2 -> [w218]
    shift-right: [w216] -> _
    shift-left: w2 -> [w217]
    tunnel: w4 -> [w215]
    shift-right: [w213] -> _
    shift-left: w1 -> [w214]
    shift-right: [w209] -> _
    shift-left: w2 -> [w211]
    shift-right: [w208] -> _
    shift-left: w2 -> [w210]
    tunnel: w3 -> [w207]
    shift-right: [w205] -> _
    shift-left: w1 -> [w206]
    stop <- w220 stop-if-true
    n126 = event shown="[0] Timeout" {
      selector: _ -> [_ _ _ _ _ _ _ _ _ _ _ _ _ _ _ _ _ _ _ _ _ _ _ _ _ _ _ _ _ _ _]
      dyn-events: _ -> [_ _ _ _ _ _ _ _ _ _ _ _ _ _ _ _ _ _ _ _ _ _ _ _ _ _ _ _ _ _ _]
      timeout: 250 -> [_ _ _ _ _ _ _ _ _ _ _ _ _ _ _ _ _ _ _ _ _ _ _ _ _ _ _ _ _ _ _]
      tunnel: [_ _ TRUE _ _ _ _ _ _ _ _ _ _ _ _ _ _ _ _ _ _ _ _ _ _ _ _ _ _ _ _] -> w220
      tunnel: w218 -> [w221 w461 w627 w659 w668 w677 w686 w698 w729 w738 w744 w757 w771 w775 w880 w889 w902 w918 w933 w939 w959 w969 w984 w991 w999 w1007 w1018 w1035 w1041 w1064 w1069]
      tunnel: w217 -> [w224 w463 w626 w658 w667 w676 w685 w697 w728 w737 w742 w755 w769 w779 w879 w888 w903 w917 w932 w938 w958 w968 w983 w992 w1000 w1006 w1017 w1034 w1039 w1063 w1072]
      tunnel: [w224 w462 w613 w658 w667 w676 w685 w697 w728 w737 w742 w755 w769 w779 w879 w888 w901 w917 w932 w938 w958 w968 w983 w992 w1000 w1006 w1017 w1034 w1039 w1063 w1072] -> w216
      tunnel: w215 -> [_ w459 _ _ _ _ _ _ _ _ _ _ _ _ _ _ _ _ _ _ _ _ _ _ _ _ _ _ _ _ _]
      tunnel: w214 -> [w227 w451 _ w657 w666 w675 w684 w694 w727 w736 w750 w762 w773 w778 w878 w890 _ w919 w931 w940 w957 w970 w980 w990 w998 w1008 w1019 w1033 w1040 w1062 w1074]
      tunnel: [w227 w453 w612 w657 w666 w675 w684 w694 w727 w736 w750 w762 w773 w778 w878 w890 w891 w919 w931 w940 w957 w970 w980 w990 w998 w1008 w1019 w1033 w1040 w1062 w1074] -> w213
      tunnel: [w222 w460 w613 w659 w668 w677 w686 w698 w729 w738 w743 w756 w770 w774 w880 w889 w904 w918 w933 w939 w959 w969 w984 w991 w999 w1007 w1018 w1035 w1041 w1064 w1068] -> w212
      tunnel: w211 -> [w226 w458 w625 w656 w665 w674 w683 w690 w726 w735 w741 w754 w768 w777 w877 w887 w900 w916 w929 w937 w956 w967 w982 w994 w1001 w1005 w1016 w1031 w1038 w1060 w1071]
      tunnel: w210 -> [w225 w457 w624 w655 w664 w673 w682 w689 w725 w734 w740 w753 w767 w776 w876 w886 w898 w915 w928 w936 w955 w966 w981 w993 w1002 w1004 w1015 w1030 w1037 w1059 w1070]
      tunnel: [w226 w456 w613 w656 w665 w674 w683 w690 w726 w735 w741 w754 w768 w777 w877 w887 w899 w916 w929 w937 w956 w967 w982 w988 w1001 w1005 w1016 w1031 w1038 w1060 w1071] -> w209
      tunnel: [w225 w455 w613 w655 w664 w673 w682 w689 w725 w734 w740 w753 w767 w776 w876 w886 w897 w915 w928 w936 w955 w966 w981 w993 w996 w1004 w1015 w1030 w1037 w1059 w1070] -> w208
      tunnel: w207 -> [_ _ w623 _ _ _ _ _ _ _ _ _ _ _ _ _ _ _ _ _ _ _ _ _ _ _ _ _ _ _ _]
      tunnel: w206 -> [w223 w454 _ w654 w663 w672 w681 w688 w724 w733 w749 w763 w772 w781 w875 w885 _ w906 w930 w935 w945 w962 w979 w987 w995 w1003 w1014 w1032 w1036 w1061 w1073]
      tunnel: [w223 w452 w612 w654 w663 w672 w681 w688 w724 w733 w749 w763 w772 w781 w875 w885 w893 w906 w930 w935 w945 w962 w979 w987 w995 w1003 w1014 w1032 w1036 w1061 w1073] -> w205
      event Timeout {
        n127 = First Call?() -> (First Call?: T/F=w228:bool)
        n128 = event-data() -> ()  [unwired: 1 in, 3 out]
        n129 = case shown="False" w228 {
          tunnel: w221 -> [w230 w394]
          tunnel: [w229 w394] -> w222
          frame False {
            n130 = stacked-sequence {
              seq-local: [w231 _ _ _] -> [_ w311 _ _]
              tunnel: w230 -> [_ _ _ w354]
              tunnel: [_ _ _ w353] -> w229
              frame #0 {
                n131 = Unbundle By Name("Log Options") -> ("Every  2"=w248:dbl, "Save to log"=w249:bool, "Every1"=w239:dbl, "Plot data"=w250:bool)
                n132 = local read "ForceSave"() -> (w240:bool)
                n133 = local read "FP Status bits"() -> (w235:u32[])
                n134 = call "Time Elapsed.vi"("Every"=w248, "Time Units"=enum16{"Minutes", "Hours", "Days"}."Minutes") -> ("Triggered?"=w244:bool)  [unwired: 1 in]
                n135 = local read "PT1 Data"() -> (w234:dbl[])
                n136 = local read "PT2 Data"() -> (w238:dbl[])
                n137 = local read "MG Data"() -> (w233:dbl[])
                n138 = call "Time Elapsed.vi"("Every"=w239, "Time Units"=enum16{"Minutes", "Hours", "Days"}."Minutes") -> ("Triggered?"=w243:bool)  [unwired: 1 in]
                n139 = local read "FP Data"() -> (w232:sgl[])
                n140 = Or(x=w240, y=w244) -> (x .or. y?=w242:bool)
                n141 = Or(x=w240, y=w243) -> (x .or. y?=w241:bool)
                n142 = And(x=w242, y=w249) -> (x .and. y?=w231:bool)
                n143 = And(x=w241, y=w250) -> (x .and. y?=w261:bool)
                n144 = case shown="True" w231 {
                  tunnel: w232 -> [_ w288]
                  tunnel: w233 -> [_ w301]
                  tunnel: w235 -> [_ w300]
                  tunnel: w234 -> [_ w302]
                  tunnel: "Log Options" -> [_ w295]
                  tunnel: w240 -> [_ _]
                  tunnel: w238 -> [_ w282]
                  frame False {
                  }
                  frame True {
                    n145 = Unbundle By Name(w295) -> ("Filename suffix"=w292:string, "AVS_Path 2"=w294:path, "AVS_FName"=w293:string, "NewFevery"=w286:u32, "Time Units"=w285:enum16{"Minutes", "Hours", "Days"}, "Date Format"=w284:string)
                    n146 = call "Combine Data 4 logging.vi"("FP Status Bits"=w300, "Time Format String"=w284, "PT2 Data"=w282, "PT1 Data"=w302, "MG Data"=w301, "FP Data"=w288) -> ("Array"=w291:string[])  [unwired: 1 in]
                    n147 = local read "Cur Path"() -> (w289:path)
                    n148 = call "Format header.vi"("FP Data"=w288) -> ("Header string"=w287:string)  [unwired: 4 in]
                    n149 = call "File Date.vi"("Cur Path"=w289) -> ("Time Stamp"=w299:timestamp)  [unwired: 4 in]
                    n150 = call "Time Elapsed time.vi"("Time Units"=w285, "Delay Time"=w286, "Time Old In"=w299) -> ("T>dT?"=w290:bool)  [unwired: 2 out]
                    n151 = case shown="True" w290 {
                      tunnel: [w304 w306] -> w297
                      tunnel: [_ w310] -> w296
                      tunnel: w294 -> [_ w309]
                      tunnel: w293 -> [_ w308]
                      tunnel: w292 -> [_ w307]
                      tunnel: w289 -> [w304 _]
                      tunnel: w287 -> [_ w305]
                      frame False {
                      }
                      frame True {
                        n152 = call "GeneratePaths.vi"("Filename Suffix"=w307, "AVS_Path"=w309, "AVS_FName"=w308) -> ("Generated Log path"=w306:path)  [unwired: 11 in, 1 out]
                        n153 = Write to Text File(file (use dialog)=w306, text=w305) -> (error out=w310:errorcluster)  [unwired: 2 in, 2 out]
                      }
                    }
                    n154 = call "Write To Spreadsheet File (string) w Error.vi"("append to file? (new file:F)"=TRUE, "error in"=w296, "1D data"=w291, "file path (dialog if empty)"=w297) -> ("new file path (Not A Path if cancelled)"=→"Cur Path":path)  [unwired: 6 in, 1 out]
                    n155 = local write "ForceSave"(FALSE ("ForceSave")) -> ()
                  }
                }
                n156 = case shown="True" w261 {
                  tunnel: w233 -> [_ w271]
                  tunnel: w232 -> [_ w281]
                  tunnel: w234 -> [_ w272]
                  tunnel: w238 -> [_ w265]
                  frame False {
                  }
                  frame True {
                    w264 = 1 ("Smoothing window")
                    n157 = Get Date/Time In Seconds() -> (seconds since 1Jan1904=w280:timestamp)
                    n158 = To Double Precision Float(number=w280) -> (double precision float=w279:dbl)
                    n159 = call "AppendData1.vi"("Smoothing window"=w264, "Current Measurement"=w279) -> ("Data Out"=w262:dbl[])  [unwired: 4 in]
                    n160 = call "AppendData.vi"("Smoothing window"=w264, "Current Measurement"=w265) -> ("Data Out"=w263:sgl[][])  [unwired: 4 in]
                    n161 = call "AppendData.vi"("Smoothing window"=w264, "Current Measurement"=w281) -> ("Data Out"=w267:sgl[][])  [unwired: 4 in]
                    n162 = call "AppendData.vi"("Smoothing window"=w264, "Current Measurement"=w271) -> ("Data Out"=w268:sgl[][])  [unwired: 4 in]
                    n163 = call "AppendData.vi"("Smoothing window"=w264, "Current Measurement"=w272) -> ("Data Out"=w269:sgl[][])  [unwired: 4 in]
                    n164 = call "MultiRPlot_Select1.vi"("Time"=w262, "FP Plots Select"="FP Plots Select", "Data In"=w267) -> ("Out Array"=→"Front Panel":cluster{"Time":dbl[], "Value":dbl[]}[])  [unwired: 1 in]
                    n165 = call "MultiRPlot_Select1.vi"("Time"=w262, "FP Plots Select"="MG Plots Select", "Data In"=w268) -> ("Out Array"=→"MaxiGauge":cluster{"Time":dbl[], "Value":dbl[]}[])  [unwired: 1 in]
                    n166 = call "MultiRPlot_Select1.vi"("Time"=w262, "FP Plots Select"="PT1 Plots Select", "Data In"=w269) -> ("Out Array"=→"PT1 Status 2":cluster{"Time":dbl[], "Value":dbl[]}[])  [unwired: 1 in]
                    n167 = call "MultiRPlot_Select1.vi"("Time"=w262, "FP Plots Select"="PT2 Plots Select", "Data In"=w263) -> ("Out Array"=→"PT2 Status":cluster{"Time":dbl[], "Value":dbl[]}[])  [unwired: 1 in]
                  }
                }
                n168 = Array To Cluster(array=w232) -> (cluster=w260:T26)
                n169 = property on="P8" class="Ring (strict)"() -> ("Value"=w258:u16)  [unwired: 2 in, 2 out]
                n170 = Unbundle(w260) -> ("FP Data[0]"=→"P1" →"P1":sgl, "FP Data[1]"=→"P2" →"P2":sgl, "FP Data[2]"=→"P3" →"P3":sgl, "FP Data[3]"=→"P4" →"P4":sgl, "FP Data[4]"=→"P5" →"P5":sgl, "FP Data[5]"=→"P6" →"4He":sgl, "FP Data[6]"=→"P7" →"3He":sgl, "FP Data[7]"=→"Flow" →"FLOW":sgl, "FP Data[8]"=→"PC" →"PC":sgl)
                n171 = Index Array(array=w233, index=w258) -> (element=→"Pstill (P8)":dbl)
              }
              frame #1 {
                n172 = case shown="True" w311 {
                  frame False {
                  }
                  frame True {
                    n173 = local read "FP Data"() -> (w316:sgl[])
                    n174 = local read "MG Data"() -> (w315:dbl[])
                    n175 = local read "PT1 Data"() -> (w314:dbl[])
                    n176 = local read "FP Status bits"() -> (w313:u32[])
                    n177 = local read "Mode"() -> (w312:u16)
                    n178 = call "FP to PGSQL.vi"("FP Data"=w316, "MG Data"=w315, "PT Data"=w314, "FP Status Bits"=w313, "Mode"=w312) -> ()  [unwired: 11 in]
                  }
                }
              }
              frame #2 {
                # "Check if the structure is \nnot empty and only one\nof Scalar or Array controls \nis set"
                # "Set FP control value from external script/program"
                n179 = local read "SetControl"() -> (w328:T7)
                n180 = Unbundle By Name(w328) -> ("Name"=w326:string, "Scalar"=w327:string, "Array"=w318:string[][])
                n181 = call <userlib>:"Empty 2D Array (String)__ogtk.vi"("Array"=w318) -> ("Empty Array?"=w321:bool)  [unwired: 8 in]
                n182 = Empty String/Path?(string/path=w326) -> (empty?=w322:bool)
                n183 = Empty String/Path?(string/path=w327) -> (empty?=w323:bool)
                n184 = Not(x=w322) -> (.not. x?=w324:bool)
                n185 = Not(x=w323) -> (.not. x?=w320:bool)
                n186 = Not(x=w321) -> (.not. x?=w317:bool)
                n187 = Exclusive Or(1:w317, 2:w320) -> (0:w319:bool)
                n188 = And(x=w324, y=w319) -> (x .and. y?=w325:bool)
                n189 = case shown="True" w325 {
                  tunnel: w326 -> [_ w332]
                  tunnel: w327 -> [_ w331]
                  tunnel: w318 -> [_ w330]
                  tunnel: w317 -> [_ w329]
                  frame False {
                  }
                  frame True {
                    n190 = flat-sequence {
                      tunnel: w332 -> [w336]
                      tunnel: w331 -> [w335]
                      tunnel: w330 -> [w333]
                      tunnel: w329 -> [w334]
                      frame #0 {
                        n191 = local read "VIRef"() -> (w337:T1)
                        n192 = case shown="True" w334 {
                          tunnel: w337 -> [w340 w343]
                          tunnel: w336 -> [w339 w342]
                          tunnel: w335 -> [w338 _]
                          tunnel: w333 -> [_ w341]
                          frame False {
                            n193 = call "Push2VI.vi"("New Value"=w338, "element"=w339, "VIRef"=w340) -> ()  [unwired: 8 in, 1 out]
                          }
                          frame True {
                            n194 = call "PushArray2VI.vi"("Str"=w341, "element"=w342, "VIRef"=w343) -> ()  [unwired: 8 in, 1 out]
                          }
                        }
                      }
                      frame #1 {
                        w345 = ""
                        # "Empty the cluster to flag that\nthe command is processed"
                        n195 = Bundle(w345, w345, "Array"=string[][] []) -> (→"SetControl":cluster{string, string, "Array":string[][]})  [unwired: 1 in]
                      }
                    }
                  }
                }
              }
              frame #3 {
                n196 = local read "MG error"() -> (w351:errorcluster)
                n197 = local read "FP error"() -> (w352:errorcluster)
                n198 = Not(x=w352) -> (.not. x?=w350:bool)
                n199 = Not(x=w351) -> (.not. x?=w349:bool)
                n200 = Compound Arithmetic op=AND(w350, w349, "EnableAutoCond") -> (w347:bool)
                n201 = case shown="True" w347 {
                  tunnel: w354 -> [w355 w371]
                  tunnel: [w355 w370] -> w353
                  frame False {
                    n202 = call <userlib>:"MGI Milliseconds Since Last Reset.vi"("Reset (F)"=TRUE) -> ()  [unwired: 5 in, 2 out]
                  }
                  frame True {
                    n203 = local read "MG Data"() -> (w378:dbl[])
                    n204 = Index Array(array=w378, index="MG  channel") -> (element=w376:dbl)
                    n205 = Not(x="Cond2") -> (.not. x?=w372:bool)
                    n206 = Less?(x=w376, y="P threshold") -> (x < y?=w374:bool)
                    n207 = Or(x=w374, y=w372) -> (x .or. y?=w358:bool)
                    "SP reached? 3" <- w358
                    n208 = Not(x=w358) -> (.not. x?=w360:bool)
                    n209 = call <userlib>:"MGI Milliseconds Since Last Reset.vi"("Reset (F)"=w360) -> ("ms"=w369:u32)  [unwired: 5 in, 1 out]
                    n210 = Divide(x=w369, y=u32 1000) -> (x/y=w366:dbl)
                    "Delay Timer" <- w366
                    n211 = Multiply(x="Delay Time", y=u32 60) -> (x*y=w362:u32)
                    n212 = Not(x="Cond1") -> (.not. x?=w363:bool)
                    n213 = Greater Or Equal?(x=w366, y=w362) -> (x >= y?=w365:bool)
                    n214 = Or(x=w365, y=w363) -> (x .or. y?=w359:bool)
                    "SP reached? 2" <- w359
                    n215 = And(x=w358, y=w359) -> (x .and. y?=w357:bool)
                    "SP reached?" <- w357
                    n216 = case shown="True" w357 {
                      tunnel: w371 -> [w379 w381]
                      tunnel: [w379 w380] -> w370
                      frame False {
                      }
                      frame True {
                        # "Auto"
                        # "Start"
                        # "Reset"
                        n217 = call "BP togglekey.vi"("keynumber"=u16 10, "FrontPanel port"=w381) -> ("error out"=w393:T18, "FrontPanel port"=w388:refnum<visa-resource-name>)  [unwired: 2 in]
                        n218 = local write "EnableAutoCond"(FALSE ("EnableAutoCond")) -> ()
                        n219 = call <userlib>:"MGI Wait (U32).vi"("ms"=u32 2000, "Error In"=w393) -> ("Error Out"=w392:errorcluster)  [unwired: 5 in]
                        n220 = call "BP togglekey.vi"("error in"=w392, "keynumber"=u16 48, "FrontPanel port"=w388) -> ("error out"=w391:T18, "FrontPanel port"=w390:refnum<visa-resource-name>)  [unwired: 1 in]
                        n221 = call <userlib>:"MGI Wait (U32).vi"("ms"=u32 500, "Error In"=w391) -> ("Error Out"=w389:errorcluster)  [unwired: 5 in]
                        n222 = call "BP togglekey.vi"("error in"=w389, "keynumber"=u16 54, "FrontPanel port"=w390) -> ("FrontPanel port"=w380:refnum<visa-resource-name>)  [unwired: 1 in, 1 out]
                      }
                    }
                  }
                }
              }
            }
          }
          frame True {
            n223 = stacked-sequence {
              frame #0 {
                w402 = T27."Page Disabled & Grayed" ("Page Enabled State")
                w403 = u8 2 ("Disabled")
                w415 = u8 1 ("Disabled")
                w419 = u32 16777062
                w424 = u32 65382
                w423 = u32 0
                w422 = 0.1
                w421 = 2000
                w420 = 0
                n224 = property class="App"() -> ("App.Kind"=w425:T28)  [unwired: 2 in, 2 out]
                n225 = property on="Hide side panel" class="Bool (strict)"("Val(Sgnl)"=FALSE ("Value (Signaling)")) -> ()  [unwired: 2 in, 2 out]
                n226 = property on="S1" class="TabCtl (strict)"("Disabled"=w403) -> ()  [unwired: 2 in, 2 out]
                n227 = property on="S2" class="TabCtl (strict)"("Disabled"=w403) -> ()  [unwired: 2 in, 2 out]
                n228 = property on="Stop" class="Bool (strict)"("Disabled"=w403) -> ()  [unwired: 2 in, 2 out]
                n229 = property on="Error panel" class="TabCtl (strict)"("Disabled"=w403) -> ()  [unwired: 2 in, 2 out]
                n230 = property on="Main Panel" class="TabCtl (strict)"("Disabled"=w403) -> ()  [unwired: 2 in, 2 out]
                n231 = property on="Main Panel" class="TabCtl (strict)"("Disabled"=w403) -> ()  [unwired: 2 in, 2 out]
                n232 = call <userlib>:"Current VIs Reference__ogtk.vi"() -> ("Current VI's reference"=w409:refnum<vi>)  [unwired: 5 in]
                n233 = case shown="\"Run Time System\"" w425 {
                  tunnel: [w427 w436] -> w426
                  frame "invalid app kind", Default {
                    n234 = control-ref of="This VI"() -> (w428:refnum<vi>)
                    n235 = property class="VI"(reference=w428) -> ("Hist.Revision"=w429:u32)  [unwired: 1 in, 2 out]
                    n236 = Divide(x=w429, y=1000.0 ("x")) -> (x/y=w433:dbl)
                    n237 = Number To Fractional String(use system decimal point (T)=FALSE, number=w433, precision (6)=i16 2) -> (F-format string=w434:string)  [unwired: 1 in]
                    n238 = Concatenate Strings("" ("string"), w434) -> (w427:string)
                  }
                  frame "Run Time System" {
                    n239 = call <userlib>:"MGI Get Executable Version.vi"() -> ("Version"=w436:string)  [unwired: 7 in]
                  }
                }
                "V" <- w426
                n240 = local write "Cur Path"(path "") -> ()
                n241 = call "GetFrontPanelControls.vi"("Ref to VI"=w409) -> ("VIRef"=w410:T1)  [unwired: 9 in, 1 out]
                "VIRef" <- w410
                n242 = Unbundle By Name(w410) -> ("Full Name"=→"ControlNames":string[])
                n243 = call <userlib>:"Current VI's Path__ogtk.vi"() -> ("Current VI's Path (+ Relative)"=w396:path)  [unwired: 1 in]
                n244 = property on="Side Panel" class="TabCtl (strict)"("Value"=enum32{"Main", "Settings", "Advanced"}."Settings" ("Side Panel")) -> ("Pages"=w399:refnum<vi>[])  [unwired: 2 in, 2 out]
                n245 = Path To String(path=w396) -> (string=→"VI path":string)
                n246 = Index Array(array=w399) -> (element #1=w400:refnum<vi>, element #3=w401:refnum<vi>)  [unwired: 3 in, 1 out]
                n247 = property class="Page"(reference=w400, "PageEnb"=w402) -> ()  [unwired: 1 in, 2 out]
                n248 = property class="Page"(reference=w401, "PageEnb"=w402) -> ()  [unwired: 1 in, 2 out]
                n249 = property on="3He" class="Slide (strict)"("Scale.Range:Minimum"=w420, "Scale.Range:Maximum"=w421, "Scale.Range:Increment"=w422) -> ()  [unwired: 2 in, 2 out]
                n250 = property on="P1" class="DigNum (strict)"("Numeric Text.Text Colors:Text Color"=w423, "Numeric Text.Text Colors:BG Color"=w419) -> ()  [unwired: 2 in, 2 out]
                n251 = property on="P4" class="DigNum (strict)"("Numeric Text.Text Colors:Text Color"=w423, "Numeric Text.Text Colors:BG Color"=w424) -> ()  [unwired: 2 in, 2 out]
                n252 = Initialize Array(FALSE, 64 ("dimension size")) -> (w395:bool[])
                n253 = property on="Start" class="Bool (strict)"("Visible"=TRUE, "Disabled"=u8 0) -> ()  [unwired: 2 in, 2 out]
                n254 = control-ref of="LEDs"() -> (w406:refnum<vi>)
                n255 = call "FP Set Binking Controls.vi"("Cluster in"=w406, "Array of blinking states"=w395, "Array of relais states"=w395) -> ()  [unwired: 13 in]
                n256 = property on="P2" class="DigNum (strict)"("Numeric Text.Text Colors:Text Color"=w423, "Numeric Text.Text Colors:BG Color"=w419) -> ()  [unwired: 2 in, 2 out]
                n257 = property on="P5" class="DigNum (strict)"("Numeric Text.Text Colors:Text Color"=w423, "Numeric Text.Text Colors:BG Color"=w424) -> ()  [unwired: 2 in, 2 out]
                n258 = property on="4He" class="Slide (strict)"("Scale.Range:Minimum"=w420, "Scale.Range:Maximum"=w421, "Scale.Range:Increment"=w422) -> ()  [unwired: 2 in, 2 out]
                n259 = control-ref of="LEDs 2"() -> (w407:refnum<vi>)
                n260 = property on="Configuration" class="Clust (strict)"("Disabled"=u8 0) -> ()  [unwired: 2 in, 2 out]
                n261 = call "FP Set Binking Controls.vi"("Cluster in"=w407, "Array of blinking states"=w395, "Array of relais states"=w395) -> ()  [unwired: 13 in]
                n262 = local write "EnableAutoCond"(FALSE ("EnableAutoCond")) -> ()
                n263 = property on="P3" class="DigNum (strict)"("Numeric Text.Text Colors:Text Color"=w423, "Numeric Text.Text Colors:BG Color"=w419) -> ()  [unwired: 2 in, 2 out]
                n264 = property on="FLOW" class="DigNum (strict)"("Numeric Text.Text Colors:Text Color"=w423, "Numeric Text.Text Colors:BG Color"=w424) -> ()  [unwired: 2 in, 2 out]
                n265 = property on="Panel ID" class="Str"("Text.Text Colors:Text Color"=u32 13311) -> ()  [unwired: 2 in, 2 out]
                n266 = property on="Buttons" class="Clust"("Disabled"=w415) -> ()  [unwired: 2 in, 2 out]
                n267 = property on="Buttons 2" class="Clust"("Disabled"=w415) -> ()  [unwired: 2 in, 2 out]
              }
              frame #1 {
                # "First load the settings from the old location then \nfrom the new one. This way the program will \"transfer\" \nthe settings to the new config file after the upgrade"
                n268 = call <userlib>:"Create Dir if Non-Existant__ogtk.vi"("Directory Path"=path "C:/LC Data/Configuration/FP" ("Relative path (.)")) -> ("dup Directory Path"=w439:path)  [unwired: 8 in, 2 out]
                n269 = call <userlib>:"Build Path - Traditional__ogtk.vi"("name or relative path"="FP config.ini", "base path"=w439) -> ("appended path"=w437:path)
                n270 = control-ref of="Configuration"() -> (w449:refnum<vi>)
                n271 = control-ref of="ADC scaling"() -> (w446:refnum<vi>)
                n272 = control-ref of="Log Options"() -> (w445:refnum<vi>)
                n273 = call <userlib>:"Current VIs Parent Directory__ogtk.vi"("Relative path (.)"=path "config.ini") -> ("Parent Directory (+ Relative)"=w447:path)  [unwired: 4 in]
                n274 = Build Array(w449, w446, w445) -> (w442:refnum<vi>[])
                n275 = call "Save Load Settings to File by Ref with path.vi"("Array of Cluster References"=w442, "Action"=enum8{"Load", "Save"}."Load", "Configuration file"=w447) -> ("error out"=w443:errorcluster)  [unwired: 6 in]
                n276 = call <userlib>:"MGI Clear Error.vi"("Error In"=w443) -> ("Error Out"=w444:errorcluster)  [unwired: 6 in]
                n277 = call "Save Load Settings to File by Ref with path.vi"("Array of Cluster References"=w442, "Action"=enum8{"Load", "Save"}."Load", "error in (no error)"=w444, "Configuration file"=w437) -> ()  [unwired: 5 in, 1 out]
              }
            }
          }
        }
      }
      event "Start": Value Change {
        n278 = event-data() -> ()  [unwired: 1 in, 6 out]
        n279 = stacked-sequence {
          tunnel: w463 -> [_ w513 _ _ _ _]
          tunnel: [_ w512 _ _ _ _] -> w462
          tunnel: w461 -> [w478 _ _ _ _ _]
          tunnel: [w465 _ _ _ _ _] -> w460
          tunnel: w459 -> [_ _ _ _ _ w611]
          tunnel: w458 -> [_ _ _ w584 _ _]
          tunnel: w457 -> [_ _ _ w583 _ _]
          tunnel: [_ _ _ w581 _ _] -> w456
          tunnel: [_ _ _ w582 _ _] -> w455
          tunnel: w451 -> [_ _ _ _ _ _]
          tunnel: w454 -> [_ _ _ _ _ _]
          tunnel: [_ _ w539 _ _ _] -> w453
          tunnel: [_ _ w543 _ _ _] -> w452
          frame #0 {
            n280 = call "Stop Display Busy AE.vi"("Action"=enum16{"Write", "Read"}."Write", "Error In"=T18 {"error"=FALSE, "code"=0, "source"=""} ("error in"), "Stop?"=FALSE) -> ("Error Out"=w466:errorcluster)  [unwired: 7 in, 1 out]
            n281 = property on="FP baud rate" class="DigNum (strict)"() -> ("Value"=w477:u32)  [unwired: 2 in, 2 out]
            n282 = call "FP-Scan ports.vi"("Error in"=w466, "baud rate"=w477, "RS232 port"=w478) -> ("Error out"=w469:errorcluster, "ID string"=w475:string, "VISA Refnum out"=w476:refnum<visa-resource-name>)  [unwired: 5 in, 1 out]
            "Panel ID" <- w475
            n283 = call "Stop Display Busy AE.vi"("Action"=enum16{"Write", "Read"}."Write", "Error In"=w469, "Stop?"=TRUE) -> ("Error Out"=w468:errorcluster)  [unwired: 7 in, 1 out]
            n284 = call "Get GHS version and type.vi"("ID string"=w475, "error in (no error)"=w468) -> ("Panel Version"=w483:bool, "System Type"=w482:bool, "error out"=w479:errorcluster)  [unwired: 4 in]
            n285 = call "Display Busy.vi"("error in (no error)"=w466, "Title"="Trying to connect to the Front Panel") -> ()  [unwired: 8 in, 2 out]
            n286 = Boolean To (0,1)(Boolean=w483) -> (0, 1=w464:i16)
            n287 = Boolean To (0,1)(Boolean=w482) -> (0, 1=w481:i16)
            n288 = property on="FP Layout" class="TabCtl (strict)"("Value"=w464) -> ()  [unwired: 2 in, 2 out]
            n289 = property on="Panel Layout" class="Enum (strict)"("Value"=w464) -> ()  [unwired: 2 in, 2 out]
            n290 = property on="Type" class="RadioBtnsControl (strict)"("Val(Sgnl)"=w481) -> ()  [unwired: 2 in, 2 out]
            n291 = call "BP query settings.vi"("error in"=w479, "FrontPanel port"=w476) -> ("error out"=w480:T18, "array of 4 x 16 bit unsigned"=w490:u16[], "FrontPanel port"=w491:refnum<visa-resource-name>)  [unwired: 2 in, 1 out]
            "FP error" <- w480
            n292 = call "BP query P5.vi"("error in"=w480, "FrontPanel port"=w491) -> ("error out"=w504:T18, "array of 2 x 16 bit unsigned"=w509:u16[], "FrontPanel port"=w510:refnum<visa-resource-name>)  [unwired: 2 in, 1 out]
            n293 = Array To Cluster(array=w490) -> (cluster=w489:T29)
            n294 = Array To Cluster(array=w509) -> (cluster=w502:T30)
            n295 = call "Disable on error.vi"("error out"=w504) -> ("Numeric"=w505:i16)
            n296 = property on="P6&7 limits" class="Clust (strict)"("Value"=w489) -> ()  [unwired: 2 in, 2 out]
            n297 = call "BP query NCP5.vi"("error in"=w480, "FrontPanel port"=w510) -> ("error out"=w507:T18, "array of 3 x 16 bit unsigned"=w508:u16[], "FrontPanel port"=w501:refnum<visa-resource-name>)  [unwired: 2 in, 1 out]
            n298 = property on="P5 Settings" class="Clust (strict)"("Value"=w502, "Disabled"=w505) -> ()  [unwired: 2 in, 2 out]
            n299 = Array To Cluster(array=w508) -> (cluster=w503:T31)
            n300 = call "Disable on error.vi"("error out"=w507) -> ("Numeric"=w506:i16)
            n301 = call "BP query NCP5B.vi"("error in"=w480, "FrontPanel port"=w501) -> ("error out"=w498:T18, "array of 3 x 16 bit unsigned"=w499:u16[], "FrontPanel port"=w500:refnum<visa-resource-name>)  [unwired: 2 in, 1 out]
            n302 = property on="NCP5 Settings" class="Clust (strict)"("Value"=w503, "Disabled"=w506) -> ()  [unwired: 2 in, 2 out]
            n303 = Array To Cluster(array=w499) -> (cluster=w496:cluster{"array of 3 x 16 bit unsigned[0]":u16})
            n304 = property on="P6&7 Settings" class="Clust (strict)"("Value"=w489) -> ()  [unwired: 2 in, 2 out]
            n305 = call "Disable on error.vi"("error out"=w498) -> ("Numeric"=w497:i16)
            n306 = call "BP Query REC.vi"("error in"=w480, "FrontPanel port"=w500) -> ("error out"=w494:T18, "array of 3 x 16 bit unsigned"=w495:u16[], "FrontPanel port"=w488:refnum<visa-resource-name>)  [unwired: 2 in, 1 out]
            n307 = property on="P5 limits" class="Clust (strict)"("Value"=w502) -> ()  [unwired: 2 in, 2 out]
            n308 = property on="NCP5B Settings" class="Clust (strict)"("Value"=w496, "Disabled"=w497) -> ()  [unwired: 2 in, 2 out]
            n309 = Array To Cluster(array=w495) -> (cluster=w492:T31)
            n310 = call "Disable on error.vi"("error out"=w494) -> ("Numeric"=w493:i16)
            n311 = call "BP Query Turbo.vi"("error in"=w480, "FrontPanel port"=w488) -> ("error out"=w486:T18, "array of 3 x 16 bit unsigned"=w485:u16[], "FrontPanel port"=w465:refnum<visa-resource-name>)  [unwired: 2 in, 1 out]
            "FP port" <- w465
            n312 = property on="REC Settings" class="Clust (strict)"("Value"=w492, "Disabled"=w493) -> ()  [unwired: 2 in, 2 out]
            n313 = property on="NCP5 limits" class="Clust (strict)"("Value"=w503) -> ()  [unwired: 2 in, 2 out]
            n314 = Array To Cluster(array=w485) -> (cluster=w484:cluster{"array of 3 x 16 bit unsigned[0]":u16})
            n315 = call "Disable on error.vi"("error out"=w486) -> ("Numeric"=w487:i16)
            n316 = property on="S1&2 Settings" class="Clust (strict)"("Value"=w484, "Disabled"=w487) -> ()  [unwired: 2 in, 2 out]
            n317 = property on="NCP5B limits" class="Clust (strict)"("Value"=w496) -> ()  [unwired: 2 in, 2 out]
            n318 = property on="REC limits" class="Clust (strict)"("Value"=w492) -> ()  [unwired: 2 in, 2 out]
            n319 = property on="FP port number" class="VISAName"("Value"=w465) -> ()  [unwired: 2 in, 2 out]
            n320 = property on="S1&2 limits" class="Clust (strict)"("Value"=w484) -> ()  [unwired: 2 in, 2 out]
          }
          frame #1 {
            w515 = T18 {"error"=FALSE, "code"=0, "source"=""}  # No error
            n321 = property on="MG Enabled?" class="Bool (strict)"() -> ("Value"=w514:bool)  [unwired: 2 in, 2 out]
            n322 = case shown="True" w514 {
              tunnel: [w518 w535] -> w511
              tunnel: [w516 w519] -> w512
              tunnel: w515 -> [w518 w525]
              tunnel: [FALSE TRUE] -> _
              tunnel: w513 -> [w516 w530]
              frame False {
                # "MaxiGauge not connected"
              }
              frame True {
                n323 = call "Stop Display Busy AE.vi"("Action"=enum16{"Write", "Read"}."Write", "Error In"=w525, "Stop?"=FALSE) -> ("Error Out"=w520:errorcluster)  [unwired: 7 in, 1 out]
                n324 = call "MG- Scan ports.vi"("Error in"=w520, "RS232 port"=w530) -> ("Error out"=w522:errorcluster, "ID string"=→"Maxigauge ID":string, "VISA Refnum out"=w529:refnum<visa-resource-name>)  [unwired: 6 in, 1 out]
                n325 = call "Stop Display Busy AE.vi"("Action"=enum16{"Write", "Read"}."Write", "Error In"=w522, "Stop?"=TRUE) -> ()  [unwired: 7 in, 2 out]
                n326 = call "Display Busy.vi"("error in (no error)"=w520, "Title"="Trying to connect to the MaxiGauge") -> ()  [unwired: 8 in, 2 out]
                n327 = call "MG Get Channels Labels.vi"("MaxiGauge port"=w529) -> ("Array"=w533:string[], "MaxiGauge port"=w519:refnum<visa-resource-name>, "error out"=w535:errorcluster)  [unwired: 1 in]
                "MG port" <- w519
                n328 = Array To Cluster(array=w533) -> (cluster=→"Cluster":T32)
                n329 = for {
                  tunnel: w533 -> [w537] mode=indexing
                  i -> [w538]
                  n330 = property on="MaxiGauge" class="XYGraph (strict)"("Active Plot"=w538, "Plot.Plot Name"=w537) -> ()  [unwired: 2 in, 2 out]
                }
                n331 = Search 1D Array(1D array=w533, element="STIL") -> (index of element=w531:i32)  [unwired: 1 in]
                n332 = property on="MG  channel P8" class="Ring (strict)"("Value"=w531) -> ()  [unwired: 2 in, 2 out]
                n333 = property on="MG port number" class="VISAName"("Value"=w519) -> ()  [unwired: 2 in, 2 out]
              }
            }
            "MG error" <- w511
          }
          frame #2 {
            n334 = property on="PT1 port \nnumber" class="VISAName"() -> ("Value"=w542:refnum<visa-resource-name>)  [unwired: 2 in, 2 out]
            n335 = property on="PT1 Enabled?" class="Bool (strict)"() -> ("Value"=w548:bool)  [unwired: 2 in, 2 out]
            n336 = case shown="True" w548 {
              tunnel: w542 -> [_ w580]
              tunnel: [u16 0 ("Port Number out") w579] -> w539
              tunnel: [errorcluster {"status"=FALSE, "code"=0, "source"=""} ("Error out") w571] -> w547
              tunnel: [refnum<visa-resource-name> refnum ("VISA Refnum out") w568] -> w540
              frame False {
              }
              frame True {
                n337 = call "Stop Display Busy AE.vi"("Action"=enum16{"Write", "Read"}."Write", "Stop?"=FALSE) -> ("Error Out"=w569:errorcluster)  [unwired: 8 in, 1 out]
                n338 = property on="PT1 Bauds" class="DigNum (strict)"() -> ("Value"=w578:u32)  [unwired: 2 in, 2 out]
                n339 = property on="PT1 Address" class="DigNum (strict)"() -> ("Value"=w577:u8)  [unwired: 2 in, 2 out]
                n340 = call "PT-Scan ports.vi"("Error in"=w569, "PT Address"=w577, "Baud rate"=w578, "RS232 port"=w580) -> ("Error out"=w572:errorcluster, "Port Number out"=w579:u16, "serial Port out"=w568:refnum<visa-resource-name>)  [unwired: 3 in, 2 out]
                n341 = call "Display Busy.vi"("error in (no error)"=w569, "Title"="Trying to connect to PulseTube1") -> ()  [unwired: 8 in, 2 out]
                n342 = property on="PT1 port \nnumber" class="VISAName"("Value"=w568) -> ()  [unwired: 2 in, 2 out]
                n343 = call "Stop Display Busy AE.vi"("Action"=enum16{"Write", "Read"}."Write", "Error In"=w572, "Stop?"=TRUE) -> ("Error Out"=w571:errorcluster)  [unwired: 7 in, 1 out]
              }
            }
            "PT1 error" <- w547
            "PT1 port" <- w539
            n344 = property on="PT2 port \nnumber" class="VISAName"() -> ("Value"=w541:refnum<visa-resource-name>)  [unwired: 2 in, 2 out]
            n345 = property on="PT2 Enabled?" class="Bool (strict)"() -> ("Value"=w545:bool)  [unwired: 2 in, 2 out]
            n346 = Build Array(w540) -> (w546:refnum<visa-resource-name>[])
            n347 = case shown="True" w545 {
              tunnel: w541 -> [_ w564]
              tunnel: [u16 0 ("Port Number out") w563] -> w543
              tunnel: [errorcluster {"status"=FALSE, "code"=0, "source"=""} ("Error out") w552] -> w544
              tunnel: w546 -> [_ w560]
              frame False {
              }
              frame True {
                n348 = call "Stop Display Busy AE.vi"("Action"=enum16{"Write", "Read"}."Write", "Stop?"=FALSE) -> ("Error Out"=w556:errorcluster)  [unwired: 8 in, 1 out]
                n349 = property on="PT2 Bauds" class="DigNum (strict)"() -> ("Value"=w562:u32)  [unwired: 2 in, 2 out]
                n350 = property on="PT2 Address" class="DigNum (strict)"() -> ("Value"=w561:u8)  [unwired: 2 in, 2 out]
                n351 = call "PT-Scan ports.vi"("RS232 ports to skip"=w560, "Error in"=w556, "PT Address"=w561, "Baud rate"=w562, "RS232 port"=w564) -> ("Error out"=w553:errorcluster, "Port Number out"=w563:u16, "serial Port out"=w551:refnum<visa-resource-name>)  [unwired: 2 in, 2 out]
                n352 = call "Display Busy.vi"("error in (no error)"=w556, "Title"="Trying to connect to PulseTube2") -> ()  [unwired: 8 in, 2 out]
                n353 = property on="PT2 port \nnumber" class="VISAName"("Value"=w551) -> ()  [unwired: 2 in, 2 out]
                n354 = call "Stop Display Busy AE.vi"("Action"=enum16{"Write", "Read"}."Write", "Error In"=w553, "Stop?"=TRUE) -> ("Error Out"=w552:errorcluster)  [unwired: 7 in, 1 out]
              }
            }
            "PT2 error" <- w544
            "PT2 port" <- w543
          }
          frame #3 {
            n355 = disable-structure shown="Disabled" {
              disable-tunnel: w584 -> [w590 w598]
              disable-tunnel: w583 -> [w589 w597]
              disable-tunnel: [w588 w597] -> w582
              disable-tunnel: [w585 w598] -> w581
              frame Disabled {
                n356 = property on="S2 Enabled?" class="Bool (strict)"() -> ("Value"=w586:bool)  [unwired: 2 in, 2 out]
                n357 = property on="S1 Enabled?" class="Bool (strict)"() -> ("Value"=w587:bool)  [unwired: 2 in, 2 out]
                n358 = case shown="False" w587 {
                  tunnel: w590 -> [w594 w596]
                  tunnel: [w594 w595] -> w585
                  frame False {
                  }
                  frame True {
                    n359 = call "PV Initialize.vi"("VISA session in"=w596) -> ("VISA session out"=w595:refnum<visa-resource-name>)  [unwired: 9 in, 1 out]
                  }
                }
                n360 = case shown="False" w586 {
                  tunnel: w589 -> [w591 w593]
                  tunnel: [w591 w592] -> w588
                  frame False {
                  }
                  frame True {
                    n361 = call "PV Initialize.vi"("VISA session in"=w593) -> ("VISA session out"=w592:refnum<visa-resource-name>)  [unwired: 9 in, 1 out]
                  }
                }
              }
              frame Enabled {
              }
            }
          }
          frame #4 {
            w600 = T27."Page Enabled" ("Page Enabled State")
            w605 = u8 0 ("Disabled")
            w608 = u8 0 ("Disabled")
            n362 = property on="Configuration" class="Clust (strict)"("Disabled"=u8 2) -> ()  [unwired: 2 in, 2 out]
            n363 = property on="Buttons" class="Clust"("Disabled"=w608) -> ()  [unwired: 2 in, 2 out]
            n364 = property on="Buttons 2" class="Clust"("Disabled"=w608) -> ()  [unwired: 2 in, 2 out]
            n365 = local write "Start"(FALSE ("Start")) -> ()
            n366 = property on="Main Panel" class="TabCtl (strict)"("Disabled"=w605) -> ()  [unwired: 2 in, 2 out]
            n367 = property on="Main Panel" class="TabCtl (strict)"("Disabled"=w605) -> ()  [unwired: 2 in, 2 out]
            n368 = property on="Stop" class="Bool (strict)"("Disabled"=w605) -> ()  [unwired: 2 in, 2 out]
            n369 = property on="Error panel" class="TabCtl (strict)"("Disabled"=w605) -> ()  [unwired: 2 in, 2 out]
            n370 = property on="Side Panel" class="TabCtl (strict)"("Value"=enum32{"Main", "Settings", "Advanced"}."Main" ("Side Panel")) -> ("Pages"=w602:refnum<vi>[])  [unwired: 2 in, 2 out]
            n371 = Index Array(array=w602) -> (element #1=w603:refnum<vi>, element #2=w599:refnum<vi>, element #3=w604:refnum<vi>)  [unwired: 3 in]
            n372 = property class="Page"(reference=w603, "PageEnb"=w600) -> ()  [unwired: 1 in, 2 out]
            n373 = property class="Page"(reference=w599, "PageEnb"=w600) -> ()  [unwired: 1 in, 2 out]
            n374 = property class="Page"(reference=w604, "PageEnb"=w600) -> ()  [unwired: 1 in, 2 out]
          }
          frame #5 {
            n375 = Set Occurrence(w611) -> ()
            n376 = property on="Start" class="Bool (strict)"("Visible"=TRUE, "Disabled"=u8 2) -> ()  [unwired: 2 in, 2 out]
          }
        }
      }
      event "Stop": Value Change {
        w612 = u16 0 ("Port Number out")
        w613 = refnum<visa-resource-name> refnum ("PT port")
        n377 = event-data() -> ()  [unwired: 1 in, 6 out]
        n378 = call "Stop Display Busy AE.vi"("Action"=enum16{"Write", "Read"}."Write", "Stop?"=FALSE) -> ("Error Out"=w616:errorcluster)  [unwired: 8 in, 1 out]
        n379 = call "Display Busy.vi"("error in (no error)"=w616, "Title"="Stopping...") -> ()  [unwired: 8 in, 2 out]
        n380 = flat-sequence {
          tunnel: w623 -> [w630]
          tunnel: [w629] -> w618
          tunnel: w616 -> [w629]
          tunnel: w627 -> [w634]
          tunnel: w626 -> [w632]
          tunnel: w625 -> [w633]
          tunnel: w624 -> [w635]
          tunnel: [w631] -> w619
          tunnel: w618 -> [w631]
          tunnel: [w638] -> w620
          tunnel: w619 -> [w638]
          tunnel: w620 -> [w645]
          tunnel: [w644] -> w615
          tunnel: w615 -> [w650]
          tunnel: [w650] -> w614
          tunnel: w614 -> [_]
          frame #0 {
            n381 = Wait on Occurrence(2:w630) -> ()  [unwired: 2 in, 1 out]
          }
          frame #1 {
            n382 = VISA Close(VISA resource name=w634) -> ()  [unwired: 1 in, 1 out]
            n383 = VISA Close(VISA resource name=w632) -> ()  [unwired: 1 in, 1 out]
            n384 = VISA Close(VISA resource name=w633) -> ()  [unwired: 1 in, 1 out]
            n385 = VISA Close(VISA resource name=w635) -> ()  [unwired: 1 in, 1 out]
          }
          frame #2 {
            n386 = control-ref of="Configuration"() -> (w641:refnum<vi>)
            n387 = control-ref of="ADC scaling"() -> (w639:refnum<vi>)
            n388 = control-ref of="Log Options"() -> (w637:refnum<vi>)
            n389 = property on="Start" class="Bool (strict)"("Visible"=TRUE) -> ()  [unwired: 2 in, 2 out]
            n390 = Build Array(w641, w639, w637) -> (w642:refnum<vi>[])
            n391 = call "Save Load Settings to File by Ref with path.vi"("Array of Cluster References"=w642, "Action"=enum8{"Load", "Save"}."Save", "Configuration file"=path "C:/LC Data/Configuration/FP/FP config.ini" ("Relative path (.)")) -> ()  [unwired: 6 in, 1 out]
          }
          frame #3 {
            n392 = call "Stop Display Busy AE.vi"("Action"=enum16{"Write", "Read"}."Write", "Error In"=w645, "Stop?"=TRUE) -> ("Error Out"=w644:errorcluster)  [unwired: 7 in, 1 out]
            n393 = property on="Stop" class="Bool (strict)"("Value"=FALSE ("stop")) -> ()  [unwired: 2 in, 2 out]
          }
          frame #4 {
            n394 = Wait (ms)(milliseconds to wait=u32 500) -> ()  [unwired: 1 out]
          }
          frame #5 {
            n395 = Stop(stop? (T)=TRUE) -> ()
          }
        }
      }
      event "PT Start": Value Change {
        w660 = u16 54529 items=["Compressor START"=54529, "Compressor STOP"=50584, "Error Code"=26020, "Reset Max/Min"=54235] ("Command")
        n396 = event-data() -> ()  [unwired: 1 in, 6 out]
        n397 = property on="PT1 Address" class="DigNum (strict)"() -> ("Value"=w653:u8)  [unwired: 2 in, 2 out]
        n398 = property on="PT1 Bauds" class="DigNum (strict)"() -> ("Value"=w652:u32)  [unwired: 2 in, 2 out]
        n399 = call "PT Send Command.vi"("PT1 port"=w657, "PT Address"=w653, "PT Bauds"=w652, "Command"=w660) -> ()  [unwired: 1 in, 2 out]
      }
      event "PT Start 2": Value Change {
        w669 = u16 54529 items=["Compressor START"=54529, "Compressor STOP"=50584, "Error Code"=26020, "Reset Max/Min"=54235] ("Command")
        n400 = event-data() -> ()  [unwired: 1 in, 6 out]
        n401 = property on="PT2 Address" class="DigNum (strict)"() -> ("Value"=w662:u8)  [unwired: 2 in, 2 out]
        n402 = property on="PT2 Bauds" class="DigNum (strict)"() -> ("Value"=w661:u32)  [unwired: 2 in, 2 out]
        n403 = call "PT Send Command.vi"("PT1 port"=w663, "PT Address"=w662, "PT Bauds"=w661, "Command"=w669) -> ()  [unwired: 1 in, 2 out]
      }
      event "PT_stop": Value Change {
        w678 = u16 50584 items=["Compressor START"=54529, "Compressor STOP"=50584, "Error Code"=26020, "Reset Max/Min"=54235] ("Command")
        n404 = event-data() -> ()  [unwired: 1 in, 1 out]
        n405 = property on="PT1 Address" class="DigNum (strict)"() -> ("Value"=w671:u8)  [unwired: 2 in, 2 out]
        n406 = property on="PT1 Bauds" class="DigNum (strict)"() -> ("Value"=w670:u32)  [unwired: 2 in, 2 out]
        n407 = call "PT Send Command.vi"("PT1 port"=w675, "PT Address"=w671, "PT Bauds"=w670, "Command"=w678) -> ()  [unwired: 1 in, 2 out]
      }
      event "PT_stop 2": Value Change {
        w687 = u16 50584 items=["Compressor START"=54529, "Compressor STOP"=50584, "Error Code"=26020, "Reset Max/Min"=54235] ("Command")
        n408 = event-data() -> ()  [unwired: 1 in, 1 out]
        n409 = property on="PT2 Address" class="DigNum (strict)"() -> ("Value"=w680:u8)  [unwired: 2 in, 2 out]
        n410 = property on="PT2 Bauds" class="DigNum (strict)"() -> ("Value"=w679:u32)  [unwired: 2 in, 2 out]
        n411 = call "PT Send Command.vi"("PT1 port"=w681, "PT Address"=w680, "PT Bauds"=w679, "Command"=w687) -> ()  [unwired: 1 in, 2 out]
      }
      event "PT Error Code": Value Change {
        n412 = event-data() -> ("OldVal"=w696:i32, "NewVal"=w692:i32)  [unwired: 1 in]
        n413 = Not Equal?(x=w696, y=w692) -> (x != y?=w695:bool)
        n414 = global read "ErrCodeStatusLkup.vi" "Error code/name/description Firmware V1.5"() -> (w693:string)
        n415 = case shown="Default" w692 {
          tunnel: w694 -> [_ w707]
          frame 0, 14..23 {
            # "No Error or Warning"
            "Attempts Counter" <- u16 0 ("Attempts Counter")
          }
          frame Default {
            # "Error"
            n416 = local read "Attempts Counter"() -> (w713:u16)
            n417 = Less?(x=w713, y="Attempts") -> (x < y?=w710:bool)
            n418 = And(x=w710, y="Restart PT on Error?") -> (x .and. y?=w709:bool)
            n419 = case shown="True" w709 {
              tunnel: "Time delay" -> [_ w715]
              tunnel: w707 -> [_ w714]
              frame False {
              }
              frame True {
                n420 = flat-sequence {
                  tunnel: w714 -> [w716]
                  tunnel: w715 -> [w720]
                  frame #0 {
                    n421 = call "PT start.vi"("PT1 port"=w716) -> ()  [unwired: 1 in, 2 out]
                  }
                  frame #1 {
                    n422 = local read "Attempts Counter"() -> (w718:u16)
                    n423 = Increment(x=w718) -> (x+1=w717:u16)
                    n424 = local write "Attempts Counter"(w717) -> ()
                  }
                  frame #2 {
                    n425 = Multiply(x=w720, y=u16 1000) -> (x*y=w721:u16)
                    n426 = Wait (ms)(milliseconds to wait=w721) -> ()  [unwired: 1 out]
                  }
                }
              }
            }
          }
        }
        n427 = Pick Line(multi-line string=w693, line index=w692) -> (output string=w691:string)  [unwired: 1 in]
        "PT Error" <- w691
        n428 = case shown="True" w695 {
          tunnel: w692 -> [_ w702]
          tunnel: w691 -> [_ w699]
          frame False {
          }
          frame True {
            n429 = Format Date/Time String() -> (date/time string=w700:string)  [unwired: 3 in]
            n430 = Number To Decimal String(number=w702) -> (decimal integer string=w701:string)  [unwired: 1 in]
            n431 = Build Array(w700, w701, w699) -> (w703:string[])
            n432 = feedback #1() -> (w704:string[][])  [unwired: 1 in]
            "Error Log" <- w704
            n433 = Build Array (concatenate)(w704, w703) -> (w705:string[][])
            n434 = feedback-in #1(w705) -> ()
          }
        }
      }
      event "PT_ResetValues": Value Change {
        w730 = u16 54235 items=["Compressor START"=54529, "Compressor STOP"=50584, "Error Code"=26020, "Reset Max/Min"=54235] ("Command")
        n435 = event-data() -> ()  [unwired: 1 in, 1 out]
        n436 = property on="PT1 Address" class="DigNum (strict)"() -> ("Value"=w723:u8)  [unwired: 2 in, 2 out]
        n437 = property on="PT1 Bauds" class="DigNum (strict)"() -> ("Value"=w722:u32)  [unwired: 2 in, 2 out]
        n438 = call "PT Send Command.vi"("PT1 port"=w727, "PT Address"=w723, "PT Bauds"=w722, "Command"=w730) -> ()  [unwired: 1 in, 2 out]
      }
      event "PT_ResetValues 2": Value Change {
        w739 = u16 54235 items=["Compressor START"=54529, "Compressor STOP"=50584, "Error Code"=26020, "Reset Max/Min"=54235] ("Command")
        n439 = event-data() -> ()  [unwired: 1 in, 1 out]
        n440 = property on="PT2 Address" class="DigNum (strict)"() -> ("Value"=w732:u8)  [unwired: 2 in, 2 out]
        n441 = property on="PT2 Bauds" class="DigNum (strict)"() -> ("Value"=w731:u32)  [unwired: 2 in, 2 out]
        n442 = call "PT Send Command.vi"("PT1 port"=w733, "PT Address"=w732, "PT Bauds"=w731, "Command"=w739) -> ()  [unwired: 1 in, 2 out]
      }
      event "Buttons": Value Change {
        n443 = event-data() -> ("NewVal"=w748:T3)  [unwired: 1 in, 5 out]
        n444 = Cluster To Array(cluster=w748) -> (array=w747:bool[])
        n445 = while {
          tunnel: w747 -> [w752] mode=indexing
          tunnel: [w751] -> w746
          i -> [w751]
          stop <- w752 stop-if-true
        }
        n446 = Increment(x=w746) -> (x+1=w745:i32)
        n447 = call "BP togglekey.vi"("keynumber"=w745, "FrontPanel port"=w744) -> ("FrontPanel port"=w743:refnum<visa-resource-name>)  [unwired: 2 in, 1 out]
      }
      event "Buttons 2": Value Change {
        n448 = event-data() -> ("NewVal"=w761:T3)  [unwired: 1 in, 5 out]
        n449 = Cluster To Array(cluster=w761) -> (array=w760:bool[])
        n450 = while {
          tunnel: w760 -> [w765] mode=indexing
          tunnel: [w764] -> w759
          i -> [w764]
          stop <- w765 stop-if-true
        }
        n451 = Increment(x=w759) -> (x+1=w758:i32)
        n452 = call "BP togglekey.vi"("keynumber"=w758, "FrontPanel port"=w757) -> ("FrontPanel port"=w756:refnum<visa-resource-name>)  [unwired: 2 in, 1 out]
      }
      event "Button": Value Change {
        n453 = event-data() -> ()  [unwired: 1 in, 6 out]
        n454 = call "BP togglekey.vi"("keynumber"="Button", "FrontPanel port"=w771) -> ("FrontPanel port"=w770:refnum<visa-resource-name>)  [unwired: 2 in, 1 out]
      }
      event "SET VALUES": Value Change {
        n455 = event-data() -> ("OldVal"=w780:bool)  [unwired: 1 in, 5 out]
        n456 = property on="SET VALUES" class="Bool (strict)"("Value"=w780) -> ()  [unwired: 2 in, 2 out]
        n457 = stacked-sequence {
          tunnel: w775 -> [w786 w800 w815 w833 w848 w863]
          tunnel: [w782 _ _ _ _ _] -> w774
          frame #0 {
            n458 = local read "P6&7 Settings"() -> (w785:T13)
            n459 = local read "P6&7 limits"() -> (w784:T13)
            n460 = Not Equal?(x=w785, y=w784) -> (x != y?=w783:bool)
            n461 = case shown="True" w783 {
              tunnel: w786 -> [w788 w795]
              tunnel: [w788 w794] -> w782
              frame False {
                n462 = control-ref of="P6&7 Settings"() -> (w787:refnum<vi>)
                n463 = call "FP check parameters error.vi"("Clust Refnum"=w787) -> ()  [unwired: 6 in, 1 out]
              }
              frame True {
                n464 = control-ref of="P6&7 Settings"() -> (w791:refnum<vi>)
                n465 = call "BP Set Config.vi"("GHS Settings"="P6&7 Settings", "FrontPanel port"=w795) -> ("error out"=w793:T18, "FrontPanel port"=w799:refnum<visa-resource-name>)  [unwired: 2 in]
                n466 = call "FP check parameters error.vi"("error in"=w793, "Clust Refnum"=w791) -> ("error out"=w792:errorcluster)  [unwired: 5 in]
                n467 = call "BP query settings.vi"("error in"=w792, "FrontPanel port"=w799) -> ("error out"=w790:T18, "array of 4 x 16 bit unsigned"=w797:u16[], "BP response"=→"Panel response":string, "FrontPanel port"=w794:refnum<visa-resource-name>)  [unwired: 2 in]
                n468 = Array To Cluster(array=w797) -> (cluster=→"P6&7 limits":T29)
                n469 = local write "FP error"(w790) -> ()
              }
            }
          }
          frame #1 {
            n470 = local read "P5 Settings"() -> (w802:cluster{"P6 low":u16, "P6 high":u16})
            n471 = local read "P5 limits"() -> (w803:cluster{"P5 C1":u16, "P5 C2":u16})
            n472 = Not Equal?(x=w802, y=w803) -> (x != y?=w801:bool)
            n473 = case shown="True" w801 {
              tunnel: w800 -> [_ w810]
              frame False {
                n474 = control-ref of="P5 Settings"() -> (w804:refnum<vi>)
                n475 = call "FP check parameters error.vi"("Clust Refnum"=w804) -> ()  [unwired: 6 in, 1 out]
              }
              frame True {
                n476 = control-ref of="P5 Settings"() -> (w807:refnum<vi>)
                n477 = call "BP Set P5.vi"("P5 Settings"="P5 Settings", "FrontPanel port in"=w810) -> ("error out"=w814:errorcluster, "FrontPanel port out"=w813:refnum<visa-resource-name>)  [unwired: 2 in]
                n478 = call "FP check parameters error.vi"("error in"=w814, "Clust Refnum"=w807) -> ("error out"=w808:errorcluster)  [unwired: 5 in]
                n479 = call "BP query P5.vi"("error in"=w808, "FrontPanel port"=w813) -> ("error out"=w806:T18, "array of 2 x 16 bit unsigned"=w812:u16[], "BP response"=w805:string)  [unwired: 2 in, 1 out]
                n480 = Array To Cluster(array=w812) -> (cluster=→"P5 limits":T30)
                n481 = local write "Panel response"(w805) -> ()
                n482 = local write "FP error"(w806) -> ()
              }
            }
          }
          frame #2 {
            n483 = local read "NCP5 Settings"() -> (w817:T10)
            n484 = local read "NCP5 limits"() -> (w818:T12)
            n485 = Not Equal?(x=w817, y=w818) -> (x != y?=w816:bool)
            n486 = case shown="True" w816 {
              tunnel: w815 -> [_ w825]
              frame False {
                n487 = control-ref of="NCP5 Settings"() -> (w819:refnum<vi>)
                n488 = call "FP check parameters error.vi"("Clust Refnum"=w819) -> ()  [unwired: 6 in, 1 out]
              }
              frame True {
                n489 = control-ref of="NCP5 Settings"() -> (w822:refnum<vi>)
                n490 = call "BP Set NCP5.vi"("NCP5 Settings"="NCP5 Settings", "FrontPanel port in"=w825) -> ("error out"=w824:errorcluster, "FrontPanel port out"=w829:refnum<visa-resource-name>)  [unwired: 2 in]
                n491 = call "FP check parameters error.vi"("error in"=w824, "Clust Refnum"=w822) -> ("error out"=w823:errorcluster)  [unwired: 5 in]
                n492 = call "BP query NCP5.vi"("error in"=w823, "FrontPanel port"=w829) -> ("error out"=w821:T18, "array of 3 x 16 bit unsigned"=w827:u16[], "BP response"=w820:string)  [unwired: 2 in, 1 out]
                n493 = local write "Panel response"(w820) -> ()
                n494 = Array To Cluster(array=w827) -> (cluster=→"NCP5 limits":T31)
                n495 = local write "FP error"(w821) -> ()
              }
            }
          }
          frame #3 {
            n496 = local read "NCP5B Settings"() -> (w830:cluster{"P6 low":u16})
            n497 = local read "NCP5B limits"() -> (w831:cluster{"P5 NC4":u16})
            n498 = Not Equal?(x=w830, y=w831) -> (x != y?=w832:bool)
            n499 = case shown="True" w832 {
              tunnel: w833 -> [_ w840]
              frame False {
                n500 = control-ref of="NCP5B Settings"() -> (w834:refnum<vi>)
                n501 = call "FP check parameters error.vi"("Clust Refnum"=w834) -> ()  [unwired: 6 in, 1 out]
              }
              frame True {
                n502 = control-ref of="NCP5B Settings"() -> (w837:refnum<vi>)
                n503 = call "BP Set NCP5B.vi"("NCP5B"="NCP5B Settings", "FrontPanel port in"=w840) -> ("error out"=w839:errorcluster, "FrontPanel port out"=w841:refnum<visa-resource-name>)  [unwired: 2 in]
                n504 = call "FP check parameters error.vi"("error in"=w839, "Clust Refnum"=w837) -> ("error out"=w838:errorcluster)  [unwired: 5 in]
                n505 = call "BP query NCP5B.vi"("error in"=w838, "FrontPanel port"=w841) -> ("error out"=w836:T18, "array of 3 x 16 bit unsigned"=w842:u16[], "BP response"=w835:string)  [unwired: 2 in, 1 out]
                n506 = local write "Panel response"(w835) -> ()
                n507 = Array To Cluster(array=w842) -> (cluster=→"NCP5B limits":cluster{"array of 3 x 16 bit unsigned[0]":u16})
                n508 = local write "FP error"(w836) -> ()
              }
            }
          }
          frame #4 {
            n509 = local read "REC Settings"() -> (w846:T10)
            n510 = local read "REC limits"() -> (w847:T11)
            n511 = Not Equal?(x=w846, y=w847) -> (x != y?=w845:bool)
            n512 = case shown="True" w845 {
              tunnel: w848 -> [_ w855]
              frame False {
                n513 = control-ref of="REC Settings"() -> (w849:refnum<vi>)
                n514 = call "FP check parameters error.vi"("Clust Refnum"=w849) -> ()  [unwired: 6 in, 1 out]
              }
              frame True {
                n515 = control-ref of="REC Settings"() -> (w852:refnum<vi>)
                n516 = call "BP Set REC.vi"("NCP5 Settings"="REC Settings", "FrontPanel port in"=w855) -> ("error out"=w854:errorcluster, "FrontPanel port out"=w856:refnum<visa-resource-name>)  [unwired: 2 in]
                n517 = call "FP check parameters error.vi"("error in"=w854, "Clust Refnum"=w852) -> ("error out"=w853:errorcluster)  [unwired: 5 in]
                n518 = call "BP Query REC.vi"("error in"=w853, "FrontPanel port"=w856) -> ("error out"=w851:T18, "array of 3 x 16 bit unsigned"=w858:u16[], "BP response"=w850:string)  [unwired: 2 in, 1 out]
                n519 = local write "Panel response"(w850) -> ()
                n520 = Array To Cluster(array=w858) -> (cluster=→"REC limits":T31)
                n521 = local write "FP error"(w851) -> ()
              }
            }
          }
          frame #5 {
            n522 = local read "S1&2 Settings"() -> (w860:cluster{"Enum":enum16{"OFF", "ON"}})
            n523 = local read "S1&2 limits"() -> (w861:cluster{"S1&S2":enum16{"OFF", "ON"}})
            n524 = Not Equal?(x=w860, y=w861) -> (x != y?=w862:bool)
            n525 = case shown="True" w862 {
              tunnel: w863 -> [_ w872]
              frame False {
                n526 = control-ref of="S1&2 Settings"() -> (w864:refnum<vi>)
                n527 = call "FP check parameters error.vi"("Clust Refnum"=w864) -> ()  [unwired: 6 in, 1 out]
              }
              frame True {
                n528 = control-ref of="S1&2 Settings"() -> (w867:refnum<vi>)
                n529 = call "BP Set Turbo.vi"("S1&2 Settings"="S1&2 Settings", "FrontPanel port in"=w872) -> ("error out"=w869:errorcluster, "FrontPanel port out"=w873:refnum<visa-resource-name>)  [unwired: 2 in]
                n530 = call "FP check parameters error.vi"("error in"=w869, "Clust Refnum"=w867) -> ("error out"=w868:errorcluster)  [unwired: 5 in]
                n531 = call "BP Query Turbo.vi"("error in"=w868, "FrontPanel port"=w873) -> ("error out"=w866:T18, "array of 3 x 16 bit unsigned"=w874:u16[], "BP response"=w865:string)  [unwired: 2 in, 1 out]
                n532 = local write "Panel response"(w865) -> ()
                n533 = Array To Cluster(array=w874) -> (cluster=→"S1&2 limits":cluster{"array of 3 x 16 bit unsigned[0]":u16})
                n534 = local write "FP error"(w866) -> ()
              }
            }
          }
        }
      }
      event "Log Options.Plot data": Value Change {
        n535 = event-data() -> ("NewVal"=w881:bool)  [unwired: 1 in, 5 out]
        n536 = property on="Main Panel" class="TabCtl (strict)"() -> ("Pages"=w884:refnum<vi>[])  [unwired: 2 in, 2 out]
        n537 = Index Array(array=w884, index=2) -> (element=w882:refnum<vi>)
        n538 = property class="Page"(reference=w882, "PageVis"=w881) -> ()  [unwired: 1 in, 2 out]
      }
      event "Autoconf": Value Change {
        n539 = event-data() -> ()  [unwired: 1 in, 6 out]
      }
      event "Configuration": Value Change {
        n540 = event-data() -> ()  [unwired: 1 in, 6 out]
        n541 = VISA Close(VISA resource name=w902) -> ()  [unwired: 1 in, 1 out]
        n542 = VISA Close(VISA resource name=w903) -> ()  [unwired: 1 in, 1 out]
        n543 = VISA Close(VISA resource name=w900) -> ()  [unwired: 1 in, 1 out]
        n544 = VISA Close(VISA resource name=w898) -> ()  [unwired: 1 in, 1 out]
        n545 = Unbundle By Name("Configuration") -> ("PT1 port number"=w892:refnum<visa-resource-name>, "PT2 port number"=w894:refnum<visa-resource-name>, "FP port number"=w904:refnum<visa-resource-name>, "MG port number"=w901:refnum<visa-resource-name>, "S1 port"=w899:refnum<visa-resource-name>, "S2 port"=w897:refnum<visa-resource-name>)
        n546 = call "VISA to RS232 Port Nr.vi"("VISA Resource Name"=w892) -> ("Port Number"=w896:u8)  [unwired: 1 in]
        n547 = call "VISA to RS232 Port Nr.vi"("VISA Resource Name"=w894) -> ("Port Number"=w895:u8)  [unwired: 1 in]
        n548 = Increment(x=w896) -> (x+1=w891:u8)
        n549 = Increment(x=w895) -> (x+1=w893:u8)
      }
      event "Type": Value Change {
        n550 = event-data() -> ("NewVal"=w909:enum32{"Wet", "CF"})  [unwired: 1 in, 5 out]
        n551 = case shown="\"CF\", Default" w909 {
          tunnel: ["COMPRESSOR" ("Label.Text") "AUX 2" ("Label.Text")] -> w914
          tunnel: [TRUE ("Visible") FALSE ("Visible")] -> w910
          tunnel: ["From\nProbe" ("Text.Text") "From\nDewar" ("Text.Text")] -> w908
          tunnel: ["From\nOVC" ("Text.Text") "From\n1K pot" ("Text.Text")] -> w907
          frame "CF", Default {
          }
          frame "Wet" {
          }
        }
        n552 = property on="Main Panel" class="TabCtl (strict)"() -> ("Pages"=w913:refnum<vi>[])  [unwired: 2 in, 2 out]
        n553 = Index Array(array=w913, index=1) -> (element=w911:refnum<vi>)
        n554 = property on="COMPR/AUX 2" class="Bool (strict)"("Caption.Text"=w914) -> ()  [unwired: 2 in, 2 out]
        n555 = property on="String 3" class="Str"("Text.Text"=w908) -> ()  [unwired: 2 in, 2 out]
        n556 = property on="String" class="Str"("Text.Text"=w907) -> ()  [unwired: 2 in, 2 out]
        n557 = property on="BYPASS" class="Bool (strict)"("Visible"=w910) -> ()  [unwired: 2 in, 2 out]
        n558 = property on="PT STATUS" class="Bool (strict)"("Visible"=w910) -> ()  [unwired: 2 in, 2 out]
        n559 = property class="Page"(reference=w911, "PageVis"=w910) -> ()  [unwired: 1 in, 2 out]
        n560 = property on="String 4" class="Str"("Text.Text"=w908) -> ()  [unwired: 2 in, 2 out]
        n561 = property on="String 2" class="Str"("Text.Text"=w907) -> ()  [unwired: 2 in, 2 out]
      }
      event "Panel Layout": Value Change {
        n562 = event-data() -> ("NewVal"=w934:enum32{"OLD", "NEW"})  [unwired: 1 in, 5 out]
        n563 = property on="FP type" class="TabCtl (strict)"("Value"=w934) -> ()  [unwired: 2 in, 2 out]
      }
      event "FP Status bits": Value Change {
        n564 = event-data() -> ("OldVal"=w943:u32[], "NewVal"=w942:u32[])  [unwired: 1 in, 4 out]
        n565 = Not Equal?(x=w943, y=w942) -> (x != y?=w941:bool)
        n566 = case shown="True" w941 {
          frame False {
          }
          frame True {
            "ForceSave" <- TRUE ("ForceSave")
          }
        }
      }
      event "Front Panel", "MaxiGauge": Shortcut Menu Activation? {
        w949 = string[] ["Log Y"] ("item names")
        w961 = string[] ["Autoscale XY"] ("item names")
        n567 = event-data() -> ("MenuRef"=w947:refnum<k9>, "CtlRef"=w946:refnum<vi>)  [unwired: 1 in]
        n568 = Insert Menu Items(4:10, 7:w961, 8:w961, 9:w947) -> (3:w948:refnum<k9>)  [unwired: 2 in, 2 out]
        n569 = property class="XYGraph (strict)"(reference=w946) -> ("YScale.Mapping Mode"=w952:u8)  [unwired: 1 in, 2 out]
        n570 = Insert Menu Items(4:13, 7:w949, 8:w949, 9:w948) -> (3:w951:refnum<k9>)  [unwired: 2 in, 2 out]
        n571 = Not Equal To 0?(x=w952) -> (x != 0?=w953:bool)
        n572 = Set Menu Item Info(6:w953, 7:"Log Y", 11:w951) -> ()  [unwired: 4 in, 2 out]
        n573 = event-data() -> ()  [unwired: 2 in, 1 out]
      }
      event "Front Panel", "MaxiGauge": Shortcut Menu Selection (User) {
        n574 = event-data() -> ("CtlRef"=w965:refnum<vi>, "ItemTag"=w971:string)  [unwired: 1 in]
        n575 = Type Cast(type=refnum<vi> refnum ("R-Plot 0"), x=w965) -> (*(type *) &x=w964:refnum<vi>)
        n576 = case shown="\"Log Y\"" w971 {
          tunnel: w964 -> [_ w972 w974]
          frame Default {
          }
          frame "Autoscale XY" {
            w973 = u8 2 ("X Scale.Scale Fit")
            n577 = property class="XYGraph (strict)"(reference=w972, "XScale.ScaleFit"=w973, "YScale.ScaleFit"=w973) -> ()  [unwired: 1 in, 2 out]
          }
          frame "Log Y" {
            n578 = property class="XYGraph (strict)"(reference=w974) -> (reference out=w975:refnum<vi>, "YScale.Mapping Mode"=w976:u8)  [unwired: 1 in, 1 out]
            n579 = Equal To 0?(x=w976) -> (x = 0?=w977:bool)
            n580 = Boolean To (0,1)(Boolean=w977) -> (0, 1=w978:i16)
            n581 = property class="XYGraph (strict)"(reference=w975, "YScale.Mapping Mode"=w978) -> ()  [unwired: 1 in, 2 out]
          }
        }
      }
      event "Front Panel", "MaxiGauge": Scale Range Change {
        w986 = u8 0 ("X Scale.Scale Fit")
        n582 = event-data() -> ("CtlRef"=w985:refnum<vi>)  [unwired: 1 in, 7 out]
        n583 = property class="XYGraph (strict)"(reference=w985, "XScale.ScaleFit"=w986, "YScale.ScaleFit"=w986) -> ()  [unwired: 1 in, 2 out]
      }
      event "Reset Error": Value Change {
        n584 = event-data() -> ()  [unwired: 1 in, 6 out]
        n585 = property on="Device address S1" class="DigNum (strict)"() -> ("Value"=w989:u8)  [unwired: 2 in, 2 out]
        n586 = call "PV Error Reset.vi"("Adress of unit"=w989, "VISA session"=w994) -> ("VISA resource out"=w988:refnum<visa-resource-name>)  [unwired: 8 in, 1 out]
      }
      event "Reset Error 2": Value Change {
        n587 = event-data() -> ()  [unwired: 1 in, 6 out]
        n588 = property on="Device address S2" class="DigNum (strict)"() -> ("Value"=w997:u8)  [unwired: 2 in, 2 out]
        n589 = call "PV Error Reset.vi"("Adress of unit"=w997, "VISA session"=w1002) -> ("VISA resource out"=w996:refnum<visa-resource-name>)  [unwired: 8 in, 1 out]
      }
      event "Configuration.S1 Enabled?": Value Change {
        n590 = event-data() -> ("NewVal"=w1013:bool)  [unwired: 1 in, 5 out]
        n591 = Not(x=w1013) -> (.not. x?=w1012:bool)
        n592 = Boolean To (0,1)(Boolean=w1012) -> (0, 1=w1011:i16)
        n593 = Multiply(x=i16 2, y=w1011) -> (x*y=w1009:i16)
        n594 = property on="S1" class="TabCtl (strict)"("Disabled"=w1009) -> ()  [unwired: 2 in, 2 out]
      }
      event "Configuration.S2 Enabled?": Value Change {
        n595 = event-data() -> ("NewVal"=w1021:bool)  [unwired: 1 in, 5 out]
        n596 = Not(x=w1021) -> (.not. x?=w1024:bool)
        n597 = Boolean To (0,1)(Boolean=w1024) -> (0, 1=w1023:i16)
        n598 = Multiply(x=i16 2, y=w1023) -> (x*y=w1020:i16)
        n599 = property on="S2" class="TabCtl (strict)"("Disabled"=w1020) -> ()  [unwired: 2 in, 2 out]
      }
      event "Configuration.PT1 Enabled?", "Configuration.PT2 Enabled?": Value Change {
        n600 = event-data() -> ()  [unwired: 1 in, 6 out]
        n601 = property on="PT1 Enabled?" class="Bool (strict)"() -> ("Value"=w1026:bool)  [unwired: 2 in, 2 out]
        n602 = property on="PT2 Enabled?" class="Bool (strict)"() -> ("Value"=w1025:bool)  [unwired: 2 in, 2 out]
        n603 = property on="Main Panel" class="TabCtl (strict)"() -> ("Pages"=w1029:refnum<vi>[])  [unwired: 2 in, 2 out]
        n604 = Or(x=w1026, y=w1025) -> (x .or. y?=w1027:bool)
        n605 = Index Array(array=w1029) -> (element #2=w1028:refnum<vi>)  [unwired: 2 in, 1 out]
        n606 = property class="Page"(reference=w1028, "PageVis"=w1027) -> ()  [unwired: 1 in, 2 out]
      }
      event "Boolean 2": Value Change {
        n607 = event-data() -> ("NewVal"=w1042:bool)  [unwired: 1 in, 5 out]
        n608 = case shown="False" w1042 {
          frame True {
            n609 = property class="VI"() -> ("Front Panel.PanelBounds"=w1043:T33)  [unwired: 2 in, 2 out]
            n610 = Unbundle By Name(w1043) -> ("Left"=w1049:i16, "Top"=w1046:i16)
            n611 = Add(x=i16 955 ("right"), y=w1049) -> (x+y=w1048:i16)
            n612 = Add(x=w1046, y=i16 730) -> (x+y=w1044:i16)
            n613 = Bundle By Name(cluster=w1043, "Right"=w1048, "Bottom"=w1044) -> (w1050:T33)
            n614 = property class="VI"("Front Panel.PanelBounds"=w1050) -> ()  [unwired: 2 in, 2 out]
          }
          frame False {
            n615 = property class="VI"() -> ("Front Panel.PanelBounds"=w1051:T33)  [unwired: 2 in, 2 out]
            n616 = Unbundle By Name(w1051) -> ("Left"=w1057:i16, "Top"=w1054:i16)
            n617 = Add(x=i16 1259 ("right"), y=w1057) -> (x+y=w1056:i16)
            n618 = Add(x=w1054, y=i16 730) -> (x+y=w1052:i16)
            n619 = Bundle By Name(cluster=w1051, "Right"=w1056, "Bottom"=w1052) -> (w1058:T33)
            n620 = property class="VI"("Front Panel.PanelBounds"=w1058) -> ()  [unwired: 2 in, 2 out]
          }
        }
      }
      event "FP Plots Select", "MG Plots Select": Value Change {
        n621 = event-data() -> ()  [unwired: 1 in, 6 out]
        n622 = local write "ForceSave"(TRUE ("ForceSave")) -> ()
      }
      event "SendCMD": Value Change {
        n623 = event-data() -> ()  [unwired: 1 in, 6 out]
        n624 = call "BP Send Command.vi"("String"="Command", "FrontPanel port in"=w1069) -> ("string after ack"=→"Response":string, "FrontPanel port out"=w1068:refnum<visa-resource-name>)  [unwired: 1 in, 1 out]
      }
    }
  }
